vi "GEA_HEWH_SM.vi"(0 "ComPort":refnum<visa-resource-name>="COM1", 1 "Destination Address":u8=96 format="%.0x", 2 "Source Address":u8=128 format="%.0x", 5 "Command":T1=15 items=["RQST_SOFTWARE_VERSION", "RQST_T2_RESISTANCE", "RQST_T3A_RESISTANCE", "RQST_T3B_RESISTANCE", "RQST_T4_RESISTANCE", "RQST_T5_RESISTANCE", "RQST_IDLB_RESISTANCE", "RQST_MODE_SELECT_RESISTANCE", "RQST_DATA_FROM_MEMORY", "RQST_DATA_FROM_DATA_FLASH", "RQST_SS_FAULT_COUNTS", "RQST_OTHER_FAULT_COUNTS", "CMD_CLEAR_FAULT_COUNTS", "RQST_HYPERTERM_OUTPUT_DATA", "CMD_RESET_FILTER_TIMES", "CMD_WRITE_SETPOINTS", "CMD_TURN_ON_OFF_DLB", "CMD_ENTER_EXIT_FCT_MODE", "CMD_SET_LEDS", "CMD_SET_EEV_DRIVE_LINES", "REQ_READ_KEY_STATUS", "RQST_READ_PERSONALITY", "CMD_ENTER_FACT_MODE", "CMD_RESET", "CMD_RESTORE_EEPROM_DEFAULTS", "CMD_SET_MODEL_NUMBER", "CMD_SET_SERIAL_NUMBER", "RQST_MODEL_NUMBER", "RQST_SERIAL_NUMBER", "CMD_TOGGLE_SERVICE_MODE", "CMD_TOGGLE_UE_SERV", "CMD_TOGGLE_LE_SERV", "CMD_REFRESH_SERVICE_TIMEOUTS", "RQST_DSM_OVERRIDE_STATUS", "RQST_STATUS_QUERY", "RQST_HEM_KWH_DATA", "RQST_SERVICE_ERROR_CODES", "RQST_OVERRIDE_STATUS", "CMD_UPDATE_DSM_LEVEL", "CMD_OVERRIDE_STATUS_CHANGED", "CMD_CLEAR_OVERRIDE_STATUS", "CMD_CLEAR_ENERGY_USAGE_CTRS", "CMD_DSM_OVERRIDES", "CMD_UPDATE_MODE", "CMD_SET_PID_P_DENOMINATOR", "CMD_SET_PID_I_DENOM_UNDER_THR", "CMD_SET_PID_I_DENOM_OVER_THR", "CMD_SET_START_POS_UNDER_THR", "CMD_SET_START_POS_OVER_THR", "CMD_SET_EEV_STOP_POSITION", "CMD_SET_AMBIENT_THRESH_1", "CMD_SET_AMBIENT_THRESH_2", "CMD_SET_AMBIENT_THRESH_3", "CMD_SET_PID_LOW_SH_TARGET", "CMD_SET_PID_MID_SH_TARGET", "RQST_PID_PARAMETERS", "CMD_COMP_OFF", "CMD_TOGGLE_FAN", "CMD_RQST_LED_STATUS", "CMD_UE_2_SECONDS", "CMD_LE_2_SECONDS", "CMD_COMP_ON", "CMD_HP_RUN_6MIN", "RQST_TEMP_RANGE", "RQST_VACATION_RANGE", "RQST_STD_ELEC_RANGE", "RQST_WATER_CAPACITY", "CMD_CANCEL_EEV_POSITION", "CMD_EEV_POSITION", "CMD_SET_CURRENTS", "RQST_SUPPORTED_MODES"], 7 "Command Data":u8[](array[numeric]) format="%02x", 9 "InitSerial?":bool=TRUE, 11 "Error In":errorcluster) -> (4 "WriteACK":bool, 6 "Read_ACK":bool, 8 "DataReturned":u8[](array[numeric]) format="%.0x", 14 "CRC Match":bool, 15 "Error Out":errorcluster)   [LabVIEW 2009]
uses:
  HEWH Command Type.ctl
  <vilib>/Instr/_visa.llb/VISA Configure Serial Port (Instr).vi
  HEWH Error Enumeration.ctl
panel:
  out "error out":errorcluster
  out "CRCRead 2":u8[](array[numeric]) format="%.0x"
  out "CRC Calc":u8[](array[numeric]) format="%.0x"
  out "CRCArray":u8[](array[numeric]) format="%.0x"
  out "Destination Read":u8 format="%.0x"
  out "Length":u8
  out "Source Read":u8 format="%.0x"
  out "Partial Message":bool
  out "Current Read Index":i32
  out "byte count":u32=40
  out "Serial Settings:Number of Bytes at Serial Port 3":u32
  out "Serial Settings:Number of Bytes at Serial Port 2":u32
  out "tStart":u32
  out "Tdiff":i32[](array[numeric])
  out "Serial Settings:Number of Bytes at Serial Port":u32
  out "Time Array":i32[](array[numeric])
  out "ACK(E1?)":u8[](array[numeric]) format="%.0x"
  out "Local?":bool
  out "State Array":string[](array[string])
  out "CRCRead":u8[](array[numeric]) format="%.0x"
  out "Command":u8[](array[numeric])=[226, 96, 8, 128, 86, 123, 137, 227] format="%.0x"
  in  "Send HEWH Cmd":bool
  in  "Write Rand":bool
  in  "Random Data":u8[](array[numeric]) format="%.0x"
  out "WriteOK":bool
  out "ReadArray":u8[](array[numeric]) format="%.0x"
  in  "OK":bool
  # "soft version 80,160\nhyerterm data 100,200"
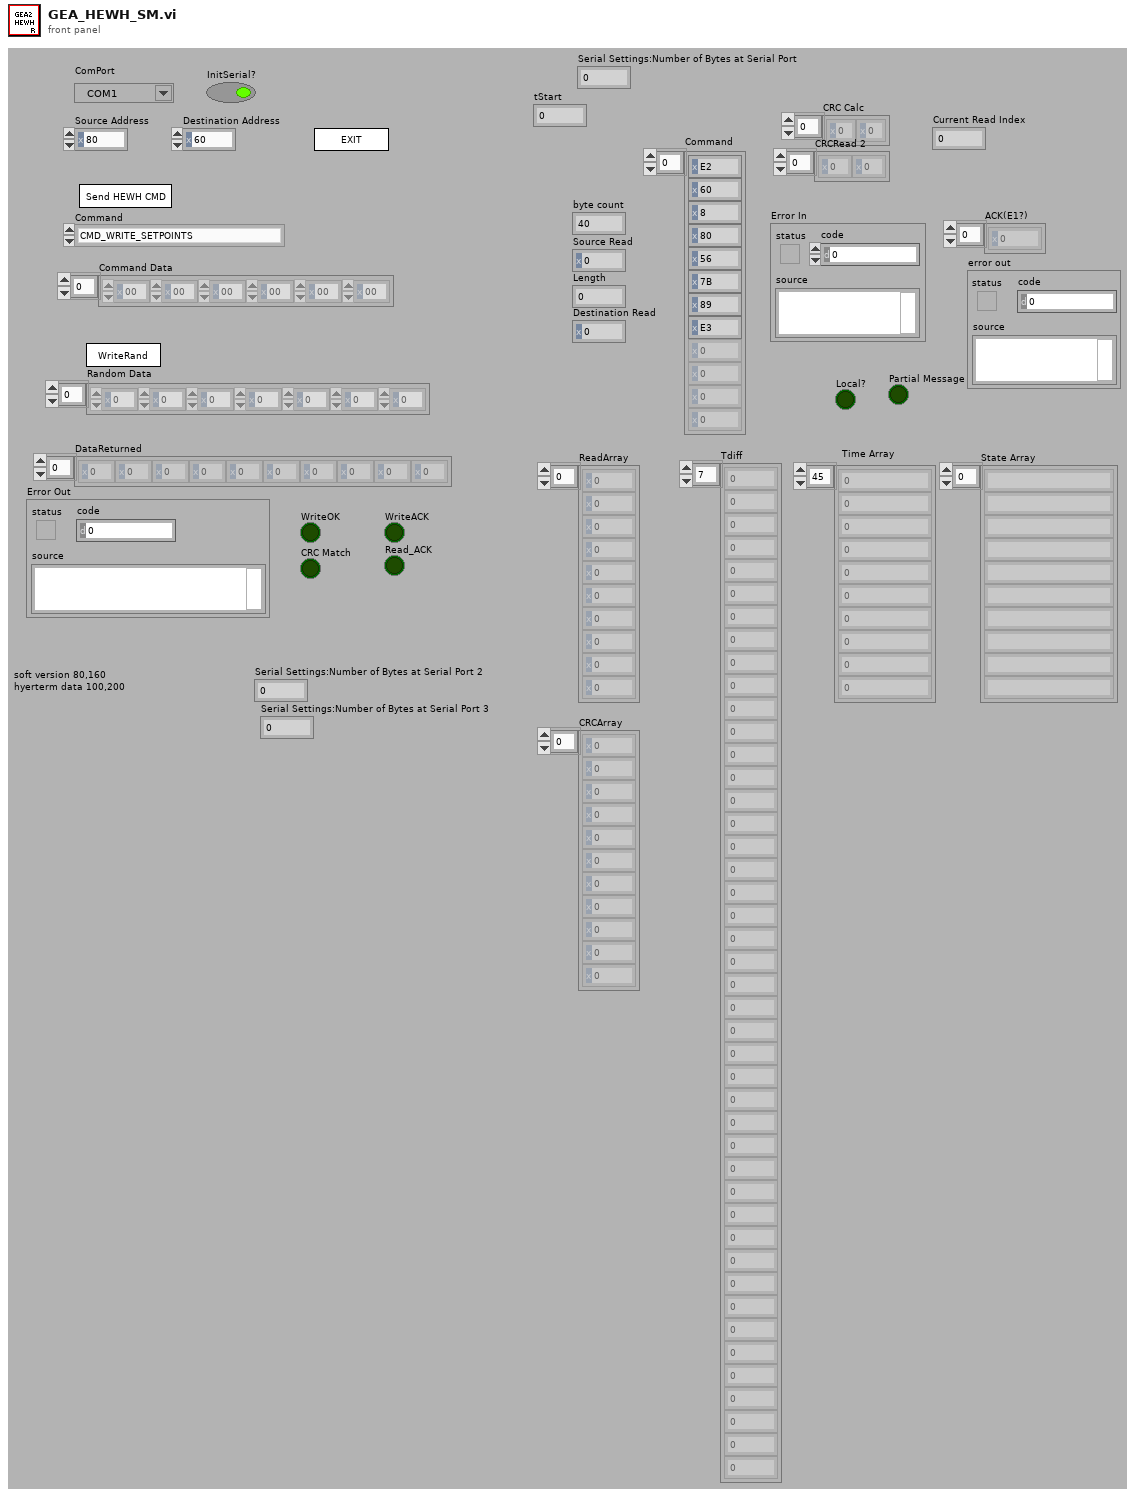
[diagram p1: front panel]
types:
  T1 = typedef "HEWH Command Type.ctl" = u8
  T2 = enum32{"invalid app kind", "Development System", "Run Time System", "Student Edition", "Embedded LabVIEW", "Evaluation", "Custom"}
  T3 = cluster{"Current VI Reference":refnum<vi>, "Close Panel on Exit?":bool}
  T4 = enum32{"Invalid", "Standard", "Closed", "Hidden", "Minimized", "Maximized"}
  T5 = typedef "HEWH Error Enumeration.ctl" = enum16{"No Error", "GEA2 Send ACK Mismatch", "GEA2 STX", "GEA2 ETX", "GEA2 CRC Mismatch", "GEA2 ReadACK", "RTD In Range Error", "Fail Mean Tank Temp", "No Flow Config Data Found", "Failed Flow During Purge", "Temp During Purge", "Confirm IF Stop Fail", "Init Draw: TC_1 Out of Range", "Flow = 0 During Draw after 20s"}
  T6 = cluster{"Core":cluster{"Current VI Reference":refnum<vi>, "Close Panel on Exit?":bool}, "ComPort":refnum<visa-resource-name>, "ReadArray":u8[], "CRCArray":u8[], "Bytes Remaining":u8, "CRCRead":u8[], "CRC":bool, "HEWH Command":u8, "Error Out Flag":bool, "Current Read Index":i32, "Total Bytes Read":u32, "Bytes Data":u8[]}
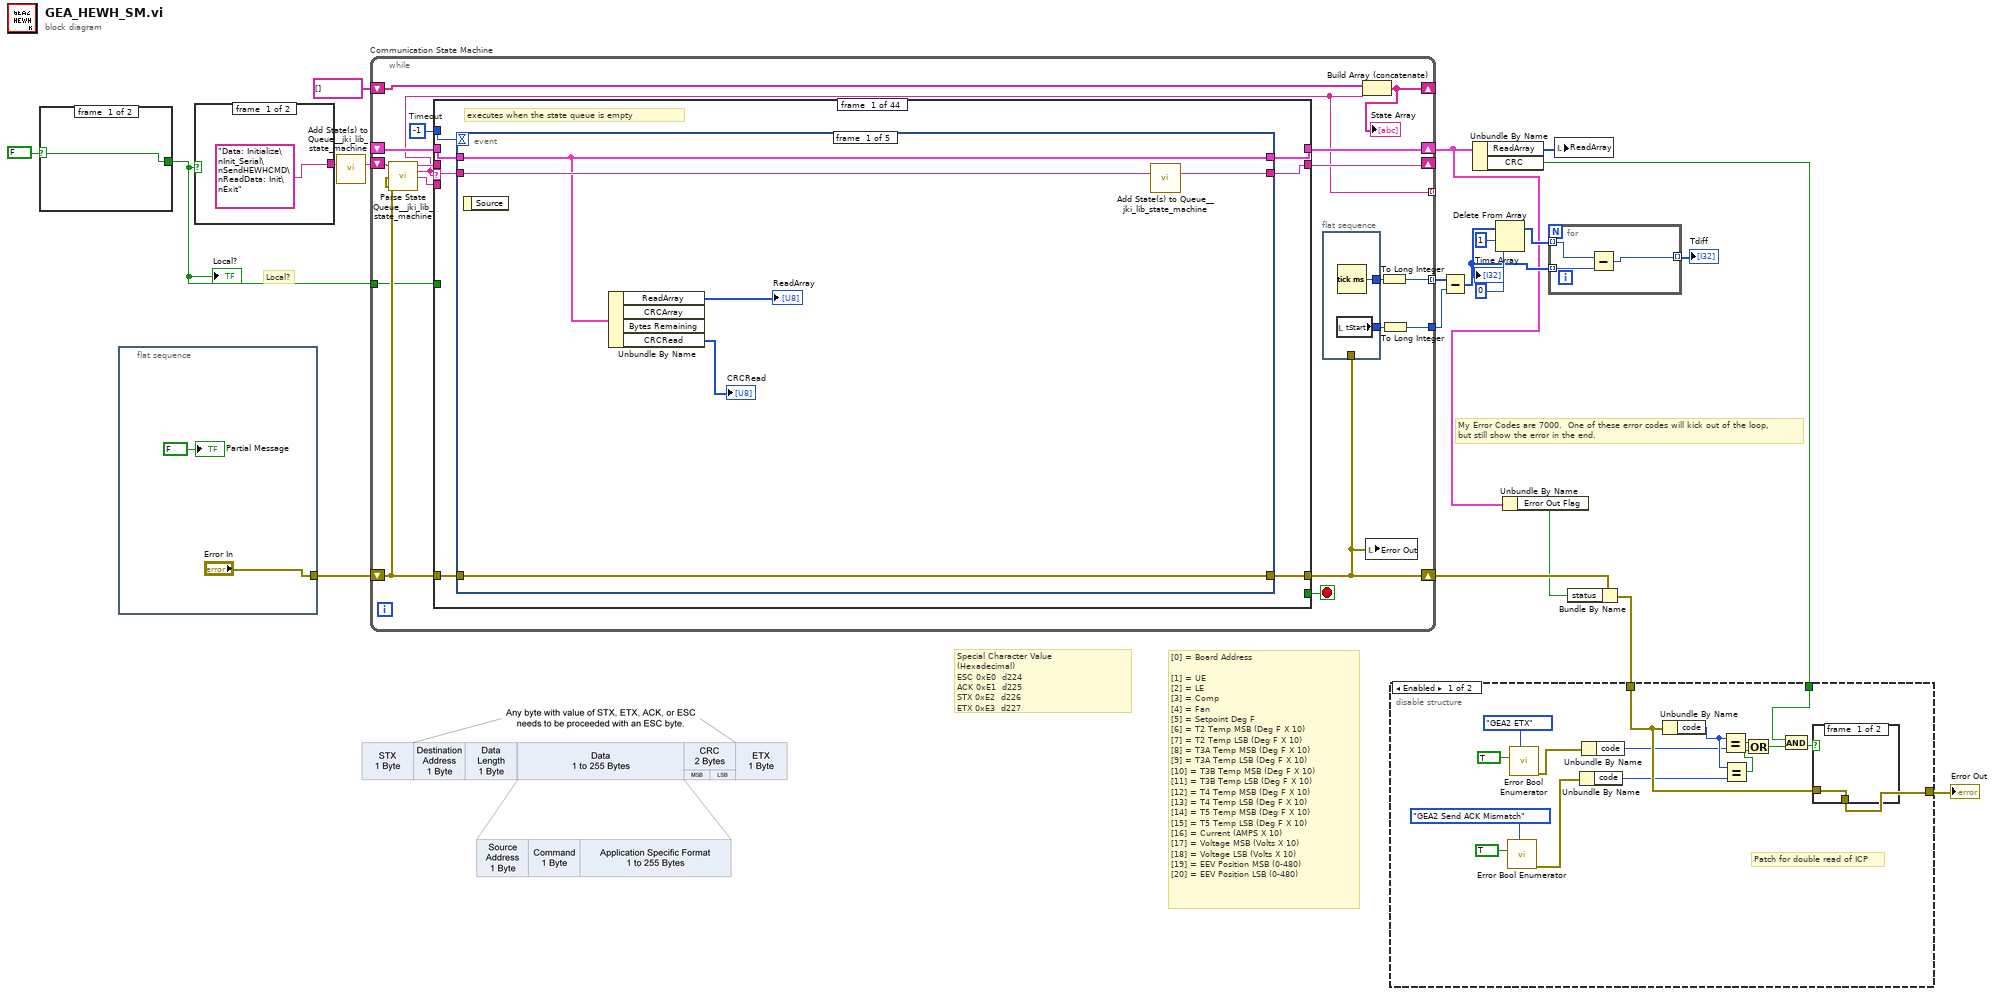
[diagram p0: block diagram]
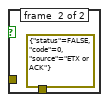
[diagram p2: hidden frame]
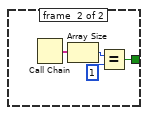
[diagram p4: hidden frame]
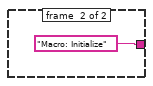
[diagram p5: hidden frame]
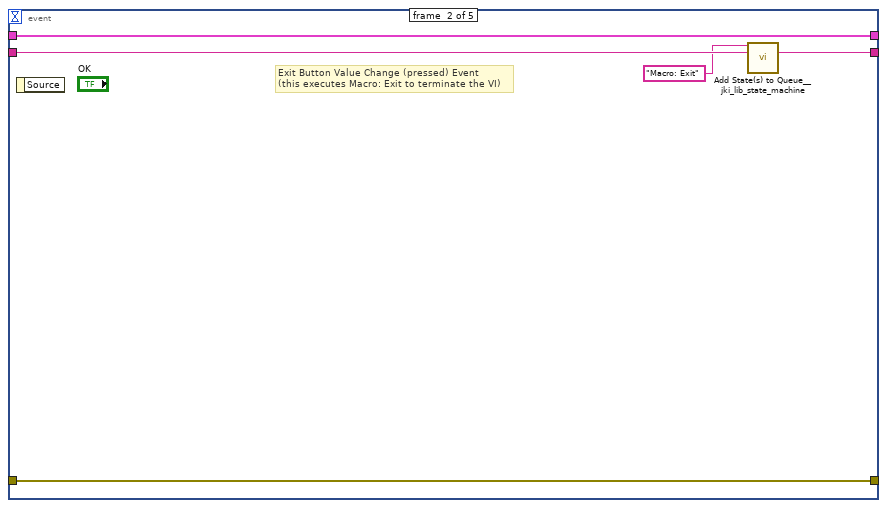
[diagram p6: hidden frame]
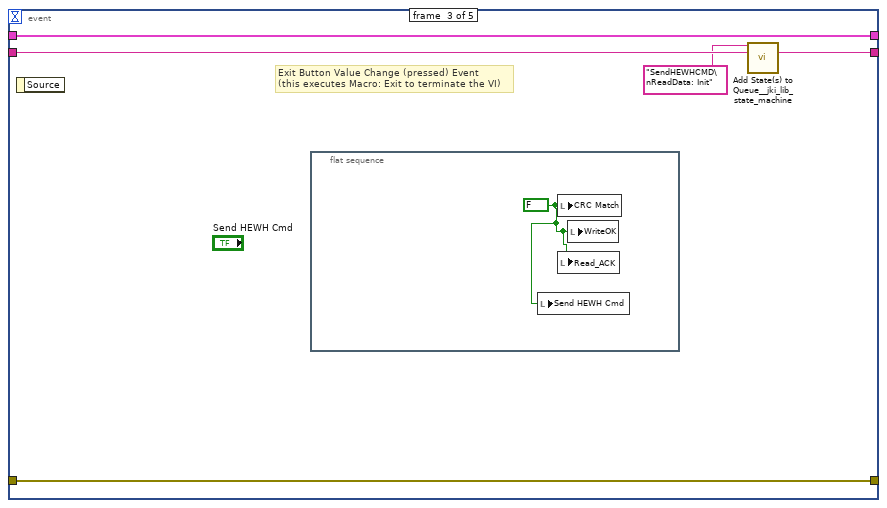
[diagram p7: hidden frame]
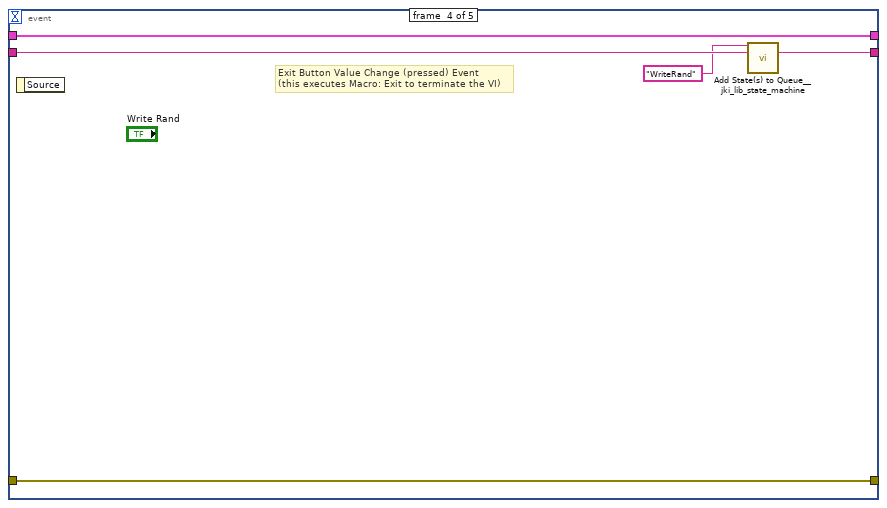
[diagram p8: hidden frame]
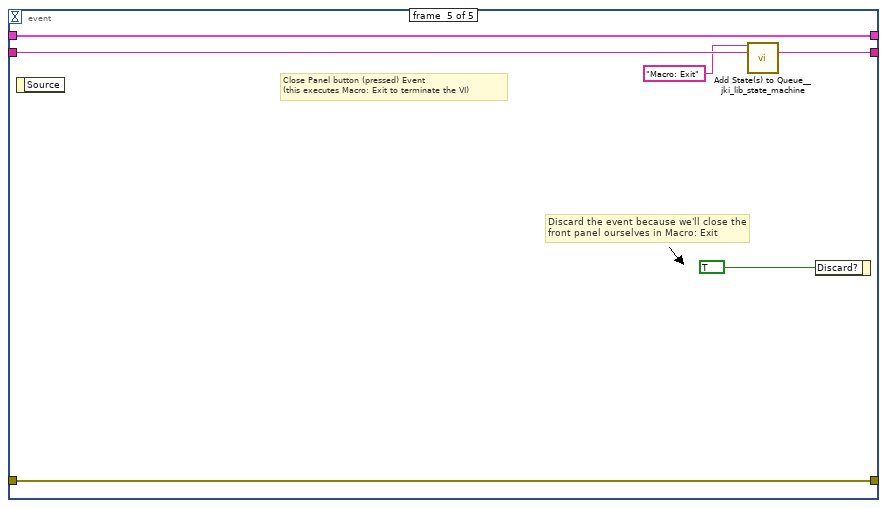
[diagram p9: hidden frame]
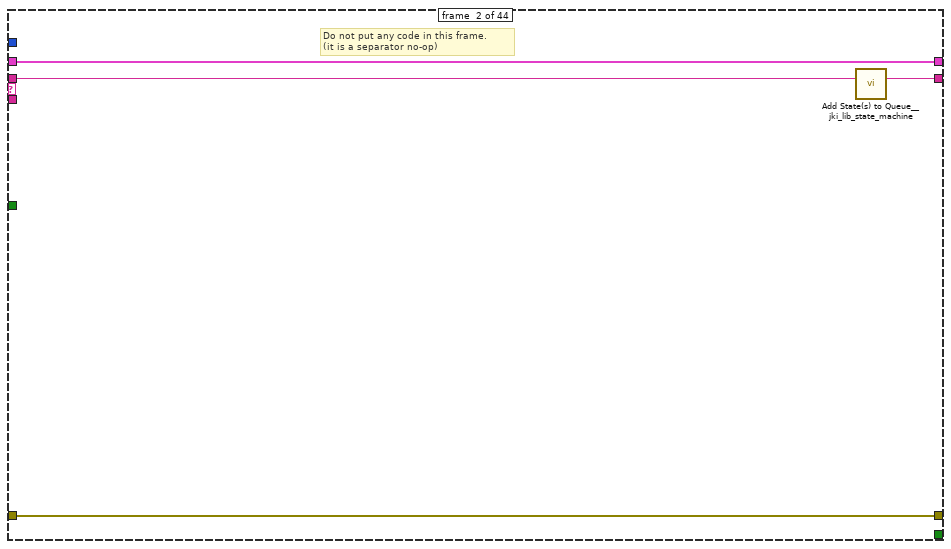
[diagram p10: hidden frame]
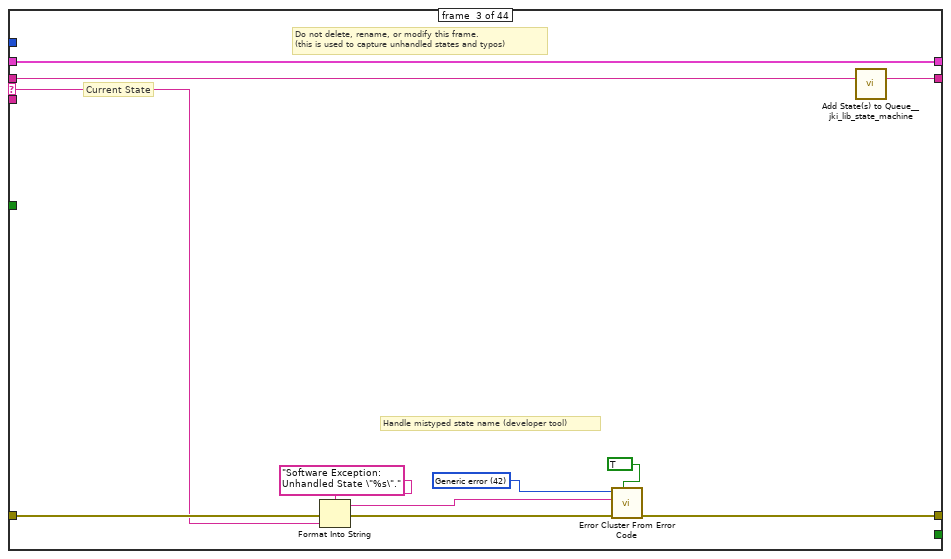
[diagram p11: hidden frame]
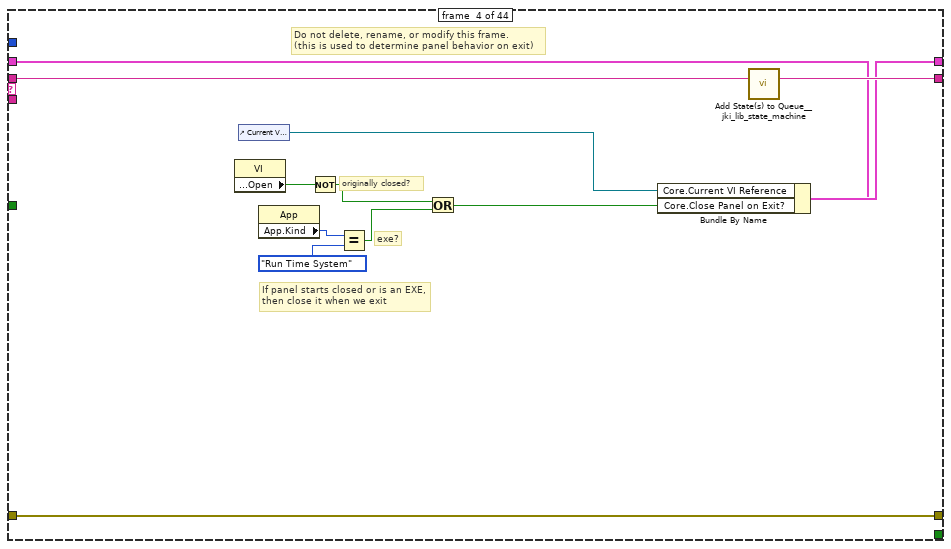
[diagram p12: hidden frame]
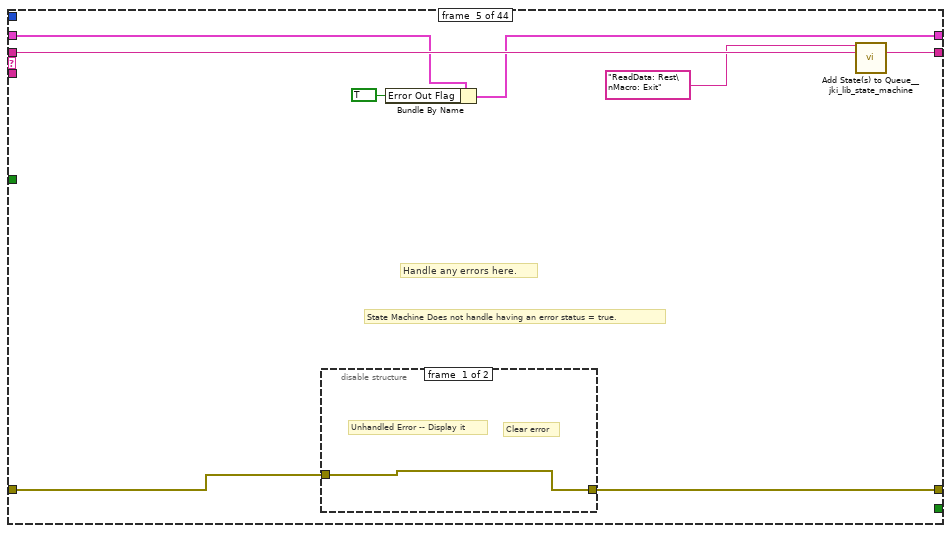
[diagram p13: hidden frame]
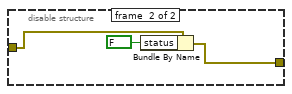
[diagram p14: hidden frame]
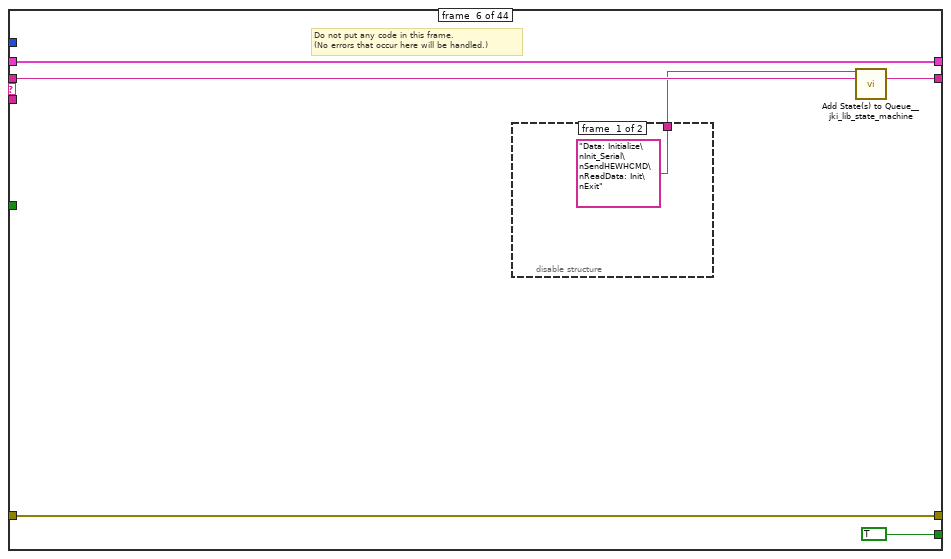
[diagram p15: hidden frame]
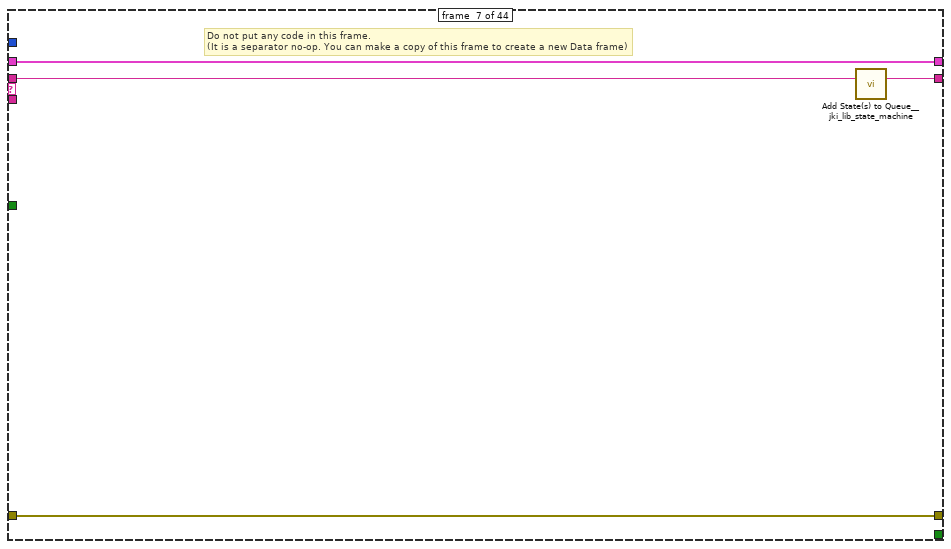
[diagram p17: hidden frame]
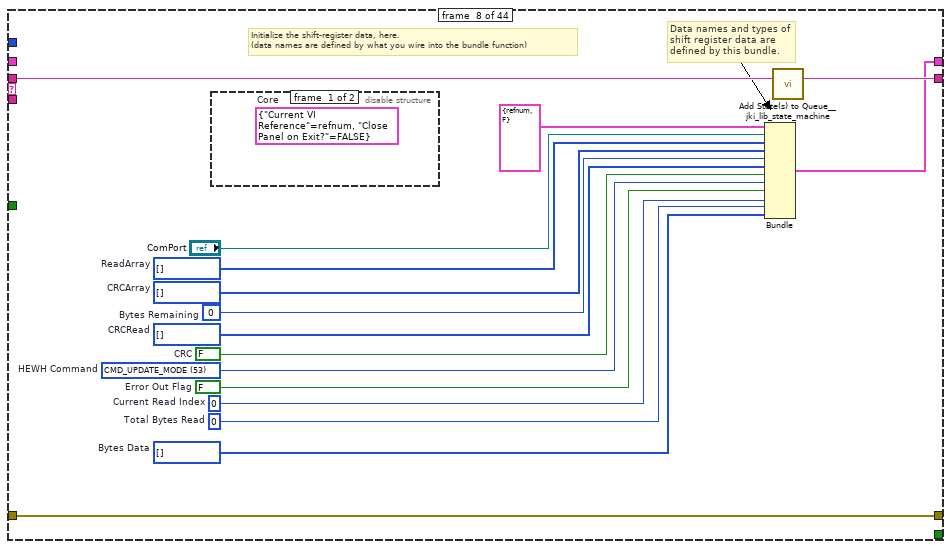
[diagram p18: hidden frame]
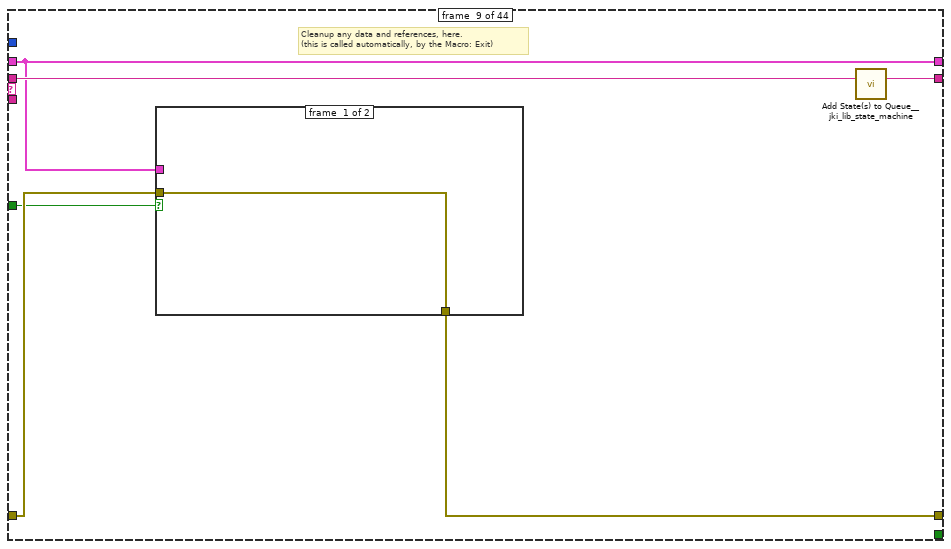
[diagram p20: hidden frame]
diagram:
  # "My Error Codes are 7000.  One of these error codes will kick out of the loop,\nbut still show the error in the end."
  # "Local?"
  # "Special Character\tValue (Hexadecimal)\nESC\t0xE0  d224\nACK\t0xE1  d225\nSTX\t0xE2  d226\nETX\t0xE3  d227"
  # "[0] = Board Address\n\n[1] = UE\n[2] = LE\n[3] = Comp\n[4] = Fan\n[5] = Setpoint Deg F\n[6] = T2 Temp MSB (Deg F X 10)\n[7] = T2 Temp LSB (Deg F X 10)\n[8] = T3A Temp MSB (Deg F X 10)\n[9] = T3A Temp LSB (Deg F X 10)\n[10] = T3B Temp MSB (Deg F X 10)\n[11] = T3B Temp LSB (Deg F X 10)\n[12] = T4 Temp MSB (Deg F X 10)\n[13] = T4 Temp LSB (Deg F X 10)\n[14] = T5 Temp MSB (Deg F X 10)\n[15] = T5 Temp LSB (Deg F X 10)\n[16] = Current (AMPS X 10)\n[17] = Voltage MSB (Volts X 10)\n[18] = Voltage LSB (Volts X 10)\n[19] = EEV Position MSB (0-480)\n[20] = EEV Position LSB (0-480)"
  n1 = case shown="False" FALSE {
    selector: FALSE -> [w21 _]
    tunnel: [w21 w22] -> w17
    frame #0 {
    }
    frame #1 {
      n2 = Call Chain() -> (call chain=w25:string[])
      n3 = Array Size(array=w25) -> (size(s)=w24:i32)
      n4 = Equal?(x=w24, y=1) -> (x = y?=w22:bool)
    }
  }
  "Local?" <- w17
  n5 = flat-sequence {
    tunnel: ["Error In"] -> w18
    frame #0 {
      "Partial Message" <- FALSE ("Partial Message")
    }
  }
  n6 = case shown="False" w17 {
    tunnel: ["Data: Initialize\nInit_Serial\nSendHEWHCMD\nReadData: Init\nExit" "Macro: Initialize"] -> w19
    frame #0 {
    }
    frame #1 {
    }
  }
  n7 = call <vilib>:"Add State(s) to Queue__jki_lib_state_machine.vi"("State(s) in (\"\")"=w19) -> ("States Out"=w20:string)  [unwired: 14 in]
  n8 = while "Communication State Machine" {
    shift-right: [w43] -> w3
    shift-left: _ -> [w42]
    shift-right: [w37] -> w16
    shift-left: w18 -> [w40]
    shift-right: [w38] -> _
    shift-left: w20 -> [w45]
    tunnel: w17 -> [w39]
    tunnel: [w31] -> _ mode=indexing
    tunnel: [w34] -> w10 mode=indexing
    tunnel: [w33] -> w9
    shift-right: [w30] -> _
    shift-left: string[] [] -> [w32]
    stop <- w44 stop-if-true
    w41 = -1  # Timeout
    n9 = call <vilib>:"Parse State Queue__jki_lib_state_machine.vi"("State Queue"=w45, "Error In (no error)"=w40) -> ("Remaining States"=w47:string, "Current State"=w31:string, "Arguments"=w46:string)  [unwired: 11 in]
    n10 = case shown="\"Error Handler\"" w31 {
      selector: w31 -> [_ _ w89 _ _ _ _ _ _ _ _ _ _ _ _ _ _ _ _ _ _ _ _ _ _ _ _ _ _ _ _ _ _ _ _ _ _ _ _ _ _ _ _ _]
      tunnel: w47 -> [w56 w88 w93 w111 w119 w129 w134 w150 w156 w165 w170 w176 w187 w213 w218 w223 w234 w243 w368 w397 w412 w422 w450 w485 w532 w576 w614 w648 w672 w699 w724 w745 w773 w779 w788 w806 w842 w869 w889 w918 w939 w960 w976 w989]
      tunnel: w46 -> [_ _ _ _ _ _ _ _ _ _ _ w171 w181 _ _ _ _ _ _ _ _ _ _ _ _ _ _ _ _ _ _ _ _ _ _ _ _ _ _ _ _ _ _ _]
      tunnel: w42 -> [w54 w85 w91 w102 w114 w127 w131 _ w153 w162 w168 w174 w183 w210 w215 w220 w231 w240 w348 w395 w409 w417 w447 w483 w529 w573 w611 w646 w663 w695 w719 w742 w753 w776 w783 w795 w829 w851 w877 w900 w927 w947 w972 w981]
      tunnel: [w53 w86 w95 w108 w117 w126 w132 w147 w151 w163 w167 w172 w184 w211 w216 w221 w232 w241 w337 w391 w410 w420 w437 w475 w522 w568 w595 w632 w667 w690 w714 w734 w756 w777 w786 w797 w840 w867 w887 w898 w937 w958 w969 w978] -> w37
      tunnel: w40 -> [w52 w86 w94 w108 w116 w126 w132 w147 w154 w163 w167 w173 w185 w211 w216 w221 w232 w238 w334 w392 w410 w420 w440 w477 w524 w569 w607 w642 w669 w693 w717 w733 w771 w777 w786 w798 w840 w867 w887 w898 w937 w958 w970 w979]
      tunnel: [w55 w87 w92 w110 w118 w128 w133 w149 w155 w164 w169 w175 w186 w212 w217 w222 w233 w242 w367 w396 w411 w421 w449 w484 w531 w575 w613 w647 w671 w698 w723 w744 w772 w778 w787 w805 w841 w868 w888 w917 w938 w959 w975 w988] -> w38
      tunnel: [_ _ _ _ _ TRUE _ _ _ _ _ _ _ _ _ _ _ _ _ _ _ _ _ _ _ _ _ _ _ _ _ _ _ _ _ _ _ _ _ _ _ _ _ _] -> w44
      tunnel: [w51 w85 w91 w109 w113 w127 w131 w148 w153 w162 w168 w174 w183 w210 w215 w220 w231 w239 w347 w395 w409 w419 w446 w482 w528 w572 w610 w645 w662 w694 w718 w741 w752 w776 w785 w794 w828 w850 w876 w899 w926 w946 w971 w980] -> w43
      tunnel: w41 -> [w50 _ _ _ _ _ _ _ _ _ _ _ _ _ _ _ _ _ _ _ _ _ _ _ _ _ _ _ _ _ _ _ _ _ _ _ _ _ _ _ _ _ _ _]
      tunnel: w39 -> [_ _ _ _ _ _ _ _ w152 _ _ _ _ _ _ _ _ w237 _ _ _ _ _ _ _ _ _ _ _ _ _ _ _ _ _ _ _ _ _ _ _ _ _ _]
      frame #0 {
        # "executes when the state queue is empty"
        n11 = event shown="[4] Panel Close?" {
          selector: _ -> [_ _ _ _ _]
          dyn-events: _ -> [_ _ _ _ _]
          timeout: w50 -> [_ _ _ _ _]
          tunnel: w56 -> [w62 w67 w72 w78 w84]
          tunnel: [w61 w66 w71 w77 w83] -> w55
          tunnel: w54 -> [w59 w64 w69 w75 w81]
          tunnel: [w60 w65 w70 w76 w82] -> w53
          tunnel: w52 -> [w60 w65 w70 w76 w82]
          tunnel: [w59 w64 w69 w75 w81] -> w51
          event #0 {
            n12 = event-data() -> ()  [unwired: 1 in, 1 out]
            n13 = Unbundle By Name(w59) -> ("ReadArray"=→"ReadArray":u8[], "CRCRead"=→"CRCRead":u8[])  [unwired: 2 out]
            n14 = call <vilib>:"Add State(s) to Queue__jki_lib_state_machine.vi"("State(s) in (\"\")"=w62) -> ("States Out"=w61:string)  [unwired: 14 in]
          }
          event #1 {
            # "Exit Button Value Change (pressed) Event\n(this executes Macro: Exit to terminate the VI)"
            n15 = event-data() -> ()  [unwired: 1 in, 1 out]
            n16 = call <vilib>:"Add State(s) to Queue__jki_lib_state_machine.vi"("State(s) in Front (\"\")"="Macro: Exit", "State(s) in (\"\")"=w67) -> ("States Out"=w66:string)  [unwired: 13 in]
          }
          event #2 {
            # "Exit Button Value Change (pressed) Event\n(this executes Macro: Exit to terminate the VI)"
            n17 = event-data() -> ()  [unwired: 1 in, 1 out]
            n18 = flat-sequence {
              frame #0 {
                w73 = FALSE ("CRC Match")
                n19 = local write "Send HEWH Cmd"(w73) -> ()
                n20 = local write "CRC Match"(w73) -> ()
                n21 = local write "Read_ACK"(w73) -> ()
                n22 = local write "WriteOK"(w73) -> ()
              }
            }
            n23 = call <vilib>:"Add State(s) to Queue__jki_lib_state_machine.vi"("State(s) in Front (\"\")"="SendHEWHCMD\nReadData: Init", "State(s) in (\"\")"=w72) -> ("States Out"=w71:string)  [unwired: 13 in]
          }
          event #3 {
            # "Exit Button Value Change (pressed) Event\n(this executes Macro: Exit to terminate the VI)"
            n24 = event-data() -> ()  [unwired: 1 in, 1 out]
            n25 = call <vilib>:"Add State(s) to Queue__jki_lib_state_machine.vi"("State(s) in Front (\"\")"="WriteRand", "State(s) in (\"\")"=w78) -> ("States Out"=w77:string)  [unwired: 13 in]
          }
          event #4 {
            # "Discard the event because we'll close the front panel ourselves in Macro: Exit"
            # "Close Panel button (pressed) Event\n(this executes Macro: Exit to terminate the VI)"
            n26 = event-data() -> ()  [unwired: 1 in, 1 out]
            n27 = call <vilib>:"Add State(s) to Queue__jki_lib_state_machine.vi"("State(s) in Front (\"\")"="Macro: Exit", "State(s) in (\"\")"=w84) -> ("States Out"=w83:string)  [unwired: 13 in]
            n28 = event-data("Discard?"=TRUE) -> ()  [unwired: 1 in, 1 out]
          }
        }
      }
      frame #1 {
        # "Do not put any code in this frame.\n(it is a separator no-op)"
        n29 = call <vilib>:"Add State(s) to Queue__jki_lib_state_machine.vi"("State(s) in (\"\")"=w88) -> ("States Out"=w87:string)  [unwired: 14 in]
      }
      frame #2 {
        w98 = 42 items=["No error", "Argument error", "Memory is full", "Out of zone", "End of file", "File already open", "Generic file I/O error", "File not found", "File permission error", "Disk is full", "Duplicate path", "Too many files open", "System feature not enabled", "Resource file not found", "Cannot add resource", "Resource not found", "Image not found", "Image memory error", "Pen does not exist", "Config type invalid", "Config token not found", "Config parse error", "Config memory error", "Bad external code format", "Bad external code offset", "External code not present", "Null window", "Destroy window error", "Null menu", "Print aborted", "Bad print record", "Print driver error", "Windows error during printing", "Memory error during printing", "Print dialog error", "Generic print error", "Invalid device refnum", "Device not found", "Device parameter error", "Device unit error", "Cannot open device", "Device call aborted", "Generic error", "Cancelled by user", "Object ID too low", "Object ID too high", "Object not in heap", "Unknown heap", "Unknown object (invalid DefProc)", "Unknown object (DefProc not in table)", "Message out of range", "Invalid (null) method", "Unknown message", "Manager call not supported", "Bad address", "Network operation in progress", "Network operation timed out", "Connection is busy", "Network attribute not supported", "Network error", "Address in use", "System out of memory", "Connection aborted", "Connection refused", "Not connected", "Already connected", "Connection closed", "Initialization error (interapplication manager)", "Bad occurrence", "Wait on unbound occurrence handler", "Occurrence queue overflow", "Datalog type conflict", "Unused", "Unrecognized type (interapplication manager)", "Memory corrupt", "Failed to make temporary DLL", "Old CIN version", "Drag socket not found", "Failed to load drop-object", "Failed to register OLE object", "Failed to release OLE object", "Format specifier type mismatch", "Unknown format specifier", "Too few format specifiers", "Too many format specifiers", "Scan failed", "Newer CIN version", "Error converting to variant", "Runtime menu error", "Password tampered", "Variant attribute not found", "Incompatible variant data type", "Event data is not available", "Event Store is not present", "Occurrence is not found", "Event Queue is not created", "Event info is not available", "Refnum passed is NULL", "Error retrieving Class GUID", "Error retrieving CoClass GUID", "Error retrieving TypeLib GUID.", "Bad built application magic bytes.", "Specific driver is different from the specific driver associated with the Logical Name.", "There is no session opened to the class driver.", "Max Error", "MAX - Error with config objects", "MAX - Error loading configuration", "MAX - Group not supported"]
        # "Current State"
        # "Do not delete, rename, or modify this frame.\n(this is used to capture unhandled states and typos)"
        # "Handle mistyped state name (developer tool)"
        n30 = Format Into String(format string="Software Exception: Unhandled State \"%s\"." ("message"), error in=w94, w89) -> (resulting string=w97:string, error out=w96:errorcluster)  [unwired: 1 in]
        n31 = call <vilib>:"Error Cluster From Error Code.vi"("show call chain? (False)"=TRUE, "error in (no error)"=w96, "error message (\"\")"=w97, "error code (0)"=w98) -> ("error out"=w95:errorcluster)  [unwired: 5 in]
        n32 = call <vilib>:"Add State(s) to Queue__jki_lib_state_machine.vi"("State(s) in (\"\")"=w93) -> ("States Out"=w92:string)  [unwired: 14 in]
      }
      frame #3 {
        # "Do not delete, rename, or modify this frame.\n(this is used to determine panel behavior on exit)"
        # "originally closed?"
        # "exe?"
        # "If panel starts closed or is an EXE, then close it when we exit"
        n33 = property class="VI"() -> ("Front Panel.Open"=w107:bool)  [unwired: 2 in, 2 out]
        n34 = control-ref of="Current VI Reference"() -> (w100:refnum<vi>)
        n35 = property class="App"() -> ("App.Kind"=w106:T2)  [unwired: 2 in, 2 out]
        n36 = Not(x=w107) -> (.not. x?=w104:bool)
        n37 = Equal?(x=w106, y=T2."Run Time System" ("Application:Kind")) -> (x = y?=w103:bool)
        n38 = Or(x=w104, y=w103) -> (x .or. y?=w101:bool)
        n39 = Bundle By Name(cluster=w102, "Core.Current VI Reference"=w100, "Core.Close Panel on Exit?"=w101) -> (w109:T6)
        n40 = call <vilib>:"Add State(s) to Queue__jki_lib_state_machine.vi"("State(s) in (\"\")"=w111) -> ("States Out"=w110:string)  [unwired: 14 in]
      }
      frame #4 {
        # "State Machine Does not handle having an error status = true."
        # "Handle any errors here."
        n41 = disable-structure shown="Enabled" {
          disable-tunnel: [w120 w122] -> w117
          disable-tunnel: w116 -> [w120 w123]
          frame #0 {
            # "Unhandled Error -- Display it"
            # "Clear error"
          }
          frame #1 {
            n42 = Bundle By Name(cluster=w123, "status"=FALSE) -> (w122:errorcluster)
          }
        }
        n43 = Bundle By Name(cluster=w114, "Error Out Flag"=TRUE) -> (w113:T6)
        n44 = call <vilib>:"Add State(s) to Queue__jki_lib_state_machine.vi"("State(s) in Front (\"\")"="ReadData: Rest\nMacro: Exit", "State(s) in (\"\")"=w119) -> ("States Out"=w118:string)  [unwired: 13 in]
      }
      frame #5 {
        # "Do not put any code in this frame.\n(No errors that occur here will be handled.)"
        n45 = disable-structure shown="Enabled" {
          disable-tunnel: ["Data: Initialize\nInit_Serial\nSendHEWHCMD\nReadData: Init\nExit" _] -> w124
          frame #0 {
          }
          frame #1 {
          }
        }
        n46 = call <vilib>:"Add State(s) to Queue__jki_lib_state_machine.vi"("State(s) in Front (\"\")"=w124, "State(s) in (\"\")"=w129) -> ("States Out"=w128:string)  [unwired: 13 in]
      }
      frame #6 {
        # "Do not put any code in this frame.\n(It is a separator no-op. You can make a copy of this frame to create a new Data frame)"
        n47 = call <vilib>:"Add State(s) to Queue__jki_lib_state_machine.vi"("State(s) in (\"\")"=w134) -> ("States Out"=w133:string)  [unwired: 14 in]
      }
      frame #7 {
        w135 = u8[] []  # Bytes Data
        w136 = u32 0  # Total Bytes Read
        w137 = 0  # Current Read Index
        w138 = FALSE  # Error Out Flag
        w139 = u8 53 items=["CMD_WRITE_SETPOINTS", "RQST_NON_CRIT_VERSION", "RQST_CRIT_VERSION", "RQST_EEPROM_VERSION", "RQST_T2_RESISTANCE", "RQST_T3A_RESISTANCE", "RQST_T3B_RESISTANCE", "RQST_T4_RESISTANCE", "RQST_T5_RESISTANCE", "RQST_IDLB_RESISTANCE", "RQST_MODE_SELECT_RESISTANCE", "RQST_STATUS INFO", "RQST_SS_FAULT_COUNTS", "RQST_OTHER_FAULT_COUNTS", "CMD_CLEAR_FAULT_COUNTS", "RQST_HYPERTERM_OUTPUT_DATA", "RQST_READ_PERSONALITY", "RQST_DSM_OVERRIDE_STATUS", "RQST_STATUS_QUERY", "RQST_HEM_KWH_DATA", "RQST_SERVICE_ERROR_CODES", "RQST_OVERRIDE_STATUS", "CMD_CLEAR_OVERRIDE_STATUS", "CMD_CLEAR_ENERGY_USAGE_CTRS", "CMD_COMP_OFF", "CMD_UE_2_SECONDS", "CMD_LE_2_SECONDS", "CMD_COMP_ON", "CMD_HP_RUN_6MIN", "RQST_TEMP_RANGE", "RQST_VACATION_RANGE", "RQST_STD_ELEC_RANGE", "RQST_WATER_CAPACITY", "CMD_CANCEL_EEV_POSITION", "RQST_SUPPORTED_MODES", "CMD_CONTROL_FAN1", "CMD_EEV_POSITION", "CMD_SET_EEV_START_POSITION", "CMD_SET_EEV_STOP_POSITION", "CMD_UPDATE_DSM_LEVEL", "CMD_SET_PID_I_DENOMINATOR", "CMD_SET_PID_I_NUMERATOR", "RQST_DATA_FROM_MEMORY", "CMD_OVERRIDE_STATUS_CHANGED", "CMD_SET_PID_P_DENOMINATOR", "CMD_SET_PID_P_NUMERATOR", "CMD_SET_PID_RUN_SH_TARGET", "CMD_SET_PID_START_DWELL_TIME", "CMD_SET_PID_TRANSITION_TIME", "CMD_SET_PID_TRANS_SH_TARGET", "CMD_SET_PID_UPDATE_RATE", "RQST_DATA_FROM_DATA_FLASH", "CMD_DSM_OVERRIDES", "CMD_UPDATE_MODE", "CMD_UPDATE_SPECIAL_OPERATION", "CMD_SET_CURRENTS", "CMD_RESET_FILTER_TIMES", "CMD_TURN_ON_DLB", "RQST_PID_PARAMETERS", "CMD_CHECK_CRC", "CMD_ENTER_FACT_MODE", "CMD_RESET", "CMD_RESTORE_EEPROM_DEFAULTS"]  # HEWH Command
        w141 = FALSE  # CRC
        w142 = u8[] []  # CRCRead
        w143 = u8 0  # Bytes Remaining
        w144 = u8[] []  # CRCArray
        w145 = u8[] []  # ReadArray
        # "Data names and types of shift register data are defined by this bundle."
        # "Initialize the shift-register data, here.\n(data names are defined by what you wire into the bundle function)"
        n48 = disable-structure shown="Enabled" {
          frame #0 {
            (unwired) T3 {"Current VI Reference"=refnum, "Close Panel on Exit?"=FALSE}  # Core
          }
          frame #1 {
          }
        }
        n49 = Bundle("Core"=T3 {"Current VI Reference"=refnum, "Close Panel on Exit?"=FALSE}, "ComPort"="ComPort", "ReadArray"=w145, "CRCArray"=w144, "Bytes Remaining"=w143, "CRCRead"=w142, "CRC"=w141, "HEWH Command"=w139, "Error Out Flag"=w138, "Current Read Index"=w137, "Total Bytes Read"=w136, "Bytes Data"=w135) -> (w148:T6)  [unwired: 1 in]
        n50 = call <vilib>:"Add State(s) to Queue__jki_lib_state_machine.vi"("State(s) in (\"\")"=w150) -> ("States Out"=w149:string)  [unwired: 14 in]
      }
      frame #8 {
        # "Cleanup any data and references, here.\n(this is called automatically, by the Macro: Exit)"
        n51 = case shown="True" w152 {
          tunnel: w154 -> [w157 w160]
          tunnel: [w157 w159] -> w151
          tunnel: w153 -> [_ w158]
          frame #0 {
          }
          frame #1 {
            n52 = Unbundle By Name(w158) -> ("Core.Current VI Reference"=w161:refnum<vi>)
            n53 = Close Reference(reference=w161, error in (no error)=w160) -> (error out=w159:errorcluster)
          }
        }
        n54 = call <vilib>:"Add State(s) to Queue__jki_lib_state_machine.vi"("State(s) in (\"\")"=w156) -> ("States Out"=w155:string)  [unwired: 14 in]
      }
      frame #9 {
        # "Do not put any code in this frame.\n(It is a separator no-op. You can make a copy of this frame to create a new UI frame)"
        n55 = call <vilib>:"Add State(s) to Queue__jki_lib_state_machine.vi"("State(s) in (\"\")"=w165) -> ("States Out"=w164:string)  [unwired: 14 in]
      }
      frame #10 {
        w166 = FALSE ("CRC Match")
        # "Initialize the User Interface, here.\n(this is called automatically, by the Macro: Init)"
        n56 = local write "CRC Match"(w166) -> ()
        n57 = local write "WriteOK"(w166) -> ()
        n58 = local write "WriteACK"(w166) -> ()
        n59 = local write "Send HEWH Cmd"(w166) -> ()
        n60 = call <vilib>:"Add State(s) to Queue__jki_lib_state_machine.vi"("State(s) in (\"\")"=w170) -> ("States Out"=w169:string)  [unwired: 14 in]
      }
      frame #11 {
        # "Argument"
        # "Set and Unset Cursor Busy.\n(Usage: \"UI: Cursor Set >> Busy|Idle\")"
        n61 = case shown="\"Idle\", Default" w171 {
          tunnel: w173 -> [w178 w180]
          tunnel: [w177 w179] -> w172
          frame #0 {
            n62 = call <vilib>:"Unset Busy.vi"("error in (no error)"=w178) -> ("error out"=w177:errorcluster)  [unwired: 10 in]
          }
          frame #1 {
            n63 = call <vilib>:"Set Busy.vi"("error in (no error)"=w180) -> ("error out"=w179:errorcluster)  [unwired: 9 in, 1 out]
          }
        }
        n64 = call <vilib>:"Add State(s) to Queue__jki_lib_state_machine.vi"("State(s) in (\"\")"=w176) -> ("States Out"=w175:string)  [unwired: 14 in]
      }
      frame #12 {
        # "Argument"
        # "Set Front Panel Open or Closed\n(Usage: \"UI: Front Panel State >> Open|Close\")"
        n65 = Unbundle By Name(w183) -> ("Core.Current VI Reference"=w182:refnum<vi>)
        n66 = case shown="\"Close\"" w181 {
          tunnel: w185 -> [w191 w204]
          tunnel: [w193 w205] -> w184
          tunnel: w182 -> [w192 w202]
          frame #0 {
            n67 = property class="VI"(reference=w192, error in=w191) -> (reference out=w189:refnum<vi>, error out=w190:errorcluster, "Front Panel.Open"=w188:bool)
            n68 = case shown="False" w188 {
              tunnel: [w196 w199] -> w193
              tunnel: w190 -> [w195 w199]
              tunnel: w189 -> [w194 _]
              frame #0 {
                n69 = invoke class="VI" method="FP.Open"(reference=w194, error in=w195, "Activate"=TRUE, "State"=T4."Standard") -> (error out=w196:errorcluster)  [unwired: 1 in, 4 out]
              }
              frame #1 {
              }
            }
          }
          frame #1 {
            n70 = property class="VI"(reference=w202, error in=w204) -> (reference out=w201:refnum<vi>, error out=w203:errorcluster, "Front Panel.Open"=w200:bool)
            n71 = case shown="True" w200 {
              tunnel: [w206 w209] -> w205
              tunnel: w203 -> [w206 w208]
              tunnel: w201 -> [_ w207]
              frame #0 {
              }
              frame #1 {
                n72 = invoke class="VI" method="FP.Close"(reference=w207, error in=w208) -> (error out=w209:errorcluster)  [unwired: 1 in, 2 out]
              }
            }
          }
        }
        n73 = call <vilib>:"Add State(s) to Queue__jki_lib_state_machine.vi"("State(s) in (\"\")"=w187) -> ("States Out"=w186:string)  [unwired: 14 in]
      }
      frame #13 {
        # "Do not put any code in this frame.\n(It is a separator no-op. You can make a copy of this frame to create a new Macro frame)"
        n74 = call <vilib>:"Add State(s) to Queue__jki_lib_state_machine.vi"("State(s) in (\"\")"=w213) -> ("States Out"=w212:string)  [unwired: 14 in]
      }
      frame #14 {
        w214 = "Data: Initialize\nInitialize Core Data\nUI: Initialize\nUI: Front Panel State >> Open\nInit_Serial"  # Data: Initialize Initialize Core Data UI: Initialize UI: Front Panel State >> Open Init_Serial
        # "Initialization Macro\n(This is called once, when the VI starts)"
        n75 = call <vilib>:"Add State(s) to Queue__jki_lib_state_machine.vi"("State(s) in Front (\"\")"=w214, "State(s) in (\"\")"=w218) -> ("States Out"=w217:string)  [unwired: 13 in]
      }
      frame #15 {
        # "Exit Macro\n(This is called once, when the VI exits)"
        n76 = disable-structure shown="Enabled" {
          disable-tunnel: w220 -> [w230 _]
          disable-tunnel: [w224 _] -> w219
          frame #0 {
            n77 = Unbundle By Name(w230) -> ("Core.Close Panel on Exit?"=w229:bool)
            n78 = Select(t="UI: Front Panel State >> Close", s=w229, f="") -> (s? t:f=w226:string)
            n79 = call <vilib>:"Add State(s) to Queue__jki_lib_state_machine.vi"("State(s) in (\"\")"=w226, "State(s) at Back (\"\")"="Data: Cleanup\nExit") -> ("States Out"=w224:string)  [unwired: 13 in]
          }
          frame #1 {
          }
        }
        n80 = call <vilib>:"Add State(s) to Queue__jki_lib_state_machine.vi"("State(s) in Front (\"\")"=w219, "State(s) in (\"\")"=w223) -> ("States Out"=w222:string)  [unwired: 13 in]
      }
      frame #16 {
        # "Template Separator\n(You can make a copy of, or modify, this frame)"
        n81 = call <vilib>:"Add State(s) to Queue__jki_lib_state_machine.vi"("State(s) in (\"\")"=w234) -> ("States Out"=w233:string)  [unwired: 14 in]
      }
      frame #17 {
        # "Your code here.\n(You can make a copy of, or modify, this frame)"
        n82 = case shown="True" "InitSerial?" {
          tunnel: [w248 w270] -> w241
          tunnel: w240 -> [w247 w280]
          tunnel: [w246 w279] -> w239
          tunnel: w238 -> [w253 w273]
          tunnel: w237 -> [_ _]
          tunnel: [w245 w271] -> w235
          frame #0 {
            # "skip error handle routine"
            n83 = Unbundle By Name(w247) -> ("ComPort"=w244:refnum<visa-resource-name>)
            n84 = property class="Instr"(reference=w244) -> (reference out=w250:refnum<visa-resource-name>, "Serial Settings:Number of Bytes at Serial Port"=w252:u32)  [unwired: 1 in, 1 out]
            n85 = Greater Than 0?(x=w252) -> (x > 0?=w251:bool)
            n86 = case shown="True" w251 {
              tunnel: w253 -> [w266 w269]
              tunnel: [w266 w268] -> w249
              tunnel: w250 -> [_ w267]
              frame #0 {
              }
              frame #1 {
                n87 = VISA Clear(VISA resource name=w267, error in (no error)=w269) -> (error out=w268:errorcluster)  [unwired: 1 out]
              }
            }
            n88 = case shown="No Error" w249 {
              selector: w249 -> [w254 w261]
              tunnel: w247 -> [w258 w265]
              tunnel: [w257 w264] -> w246
              tunnel: w244 -> [w256 _]
              tunnel: ["" ("State(s) in Front (\"\")") "Macro: Exit" ("State(s) in Front (\"\")")] -> w245
              tunnel: [w254 w260] -> w248
              frame #0 {
                n89 = Bundle By Name(cluster=w258, "ComPort"=w256) -> (w257:T6)
              }
              frame #1 {
                n90 = Bundle By Name(cluster=w265, "Error Out Flag"=TRUE) -> (w264:T6)
                n91 = Bundle By Name(cluster=w261, "status"=FALSE) -> (w260:errorcluster)
              }
            }
          }
          frame #1 {
            # "skip error handle routine"
            # "Assumes that if the serial port is 19200, then it is all ok."
            n92 = Unbundle By Name(w280) -> ("ComPort"=w278:refnum<visa-resource-name>)
            n93 = disable-structure shown="Enabled" {
              disable-tunnel: w278 -> [w316 _]
              disable-tunnel: [w313 TRUE] -> w277
              frame #0 {
                n94 = property class="Instr"(reference=w316) -> ("Baud"=w315:u32)  [unwired: 1 in, 2 out]
                n95 = Not Equal?(x=w315, y=u32 19200) -> (x != y?=w313:bool)
              }
              frame #1 {
              }
            }
            n96 = case shown="True" w277 {
              tunnel: [w318 w321] -> w276
              tunnel: [w319 w320] -> w274
              tunnel: w273 -> [w318 w323]
              tunnel: w278 -> [w319 w322]
              frame #0 {
              }
              frame #1 {
                w329 = u16 0 items=["None", "XON/XOFF", "RTS/CTS", "XON/XOFF & RTS/CTS", "DTR/DSR", "XON/XOFF & DTR/DSR"] ("flow control (0:none)")
                w328 = u16 10 items=["1.0"=10, "1.5"=15, "2.0"=20] ("stop bits (10: 1 bit)")
                n97 = call-poly "VISA Configure Serial Port"("VISA resource name"=w322, "timeout (10sec)"=u32 1000, "Enable Termination\nChar (T)"=FALSE ("Enable Termination\nChar (T)"), "baud rate (9600)"=u32 19200, "data bits (8)"=u16 8, "parity (0:none)"=enum16{"None", "Odd", "Even", "Mark", "Space"}."None", "error in (no error)"=w323, "stop bits (10: 1 bit)"=w328, "flow control (0:none)"=w329) -> ("VISA resource name out"=w320:refnum<visa-resource-name>, "error out"=w321:errorcluster)  [unwired: 5 in]
              }
            }
            n98 = disable-structure shown="Enabled" {
              disable-tunnel: w276 -> [w298 w312]
              disable-tunnel: [w297 w311] -> w272
              disable-tunnel: [w296 w310] -> w275
              disable-tunnel: w274 -> [w295 w310]
              frame #0 {
                n99 = disable-structure shown="Enabled" {
                  disable-tunnel: w295 -> [w301 w303]
                  disable-tunnel: [w300 w303] -> w294
                  disable-tunnel: [w299 u32 1 ("Bytes at Port")] -> w293
                  frame #0 {
                    n100 = property class="Instr"(reference=w301) -> (reference out=w300:refnum<visa-resource-name>, "Serial Settings:Number of Bytes at Serial Port"=w299:u32)  [unwired: 1 in, 1 out]
                  }
                  frame #1 {
                  }
                }
                n101 = case shown="1, Default" w293 {
                  tunnel: w298 -> [w305 w309]
                  tunnel: [w305 w308] -> w297
                  tunnel: [w304 w307] -> w296
                  tunnel: w294 -> [w304 w306]
                  frame #0 {
                  }
                  frame #1 {
                    n102 = VISA Clear(VISA resource name=w306, error in (no error)=w309) -> (VISA resource name out=w307:refnum<visa-resource-name>, error out=w308:errorcluster)
                  }
                }
              }
              frame #1 {
                n103 = VISA Flush I/O Buffer(VISA resource name=w310, error in (no error)=w312) -> (error out=w311:errorcluster)  [unwired: 1 in, 1 out]
              }
            }
            n104 = case shown="Error" w272 {
              selector: w272 -> [w281 w288]
              tunnel: w280 -> [w285 w292]
              tunnel: [w284 w291] -> w279
              tunnel: w275 -> [w283 _]
              tunnel: ["" ("State(s) in Front (\"\")") "Macro: Exit" ("State(s) in Front (\"\")")] -> w271
              tunnel: [w281 w286] -> w270
              frame #0 {
                n105 = Bundle By Name(cluster=w285, "ComPort"=w283) -> (w284:T6)
              }
              frame #1 {
                n106 = Bundle By Name(cluster=w292, "Error Out Flag"=TRUE) -> (w291:T6)
                n107 = Bundle By Name(cluster=w288, "status"=FALSE) -> (w286:errorcluster)
              }
            }
          }
        }
        n108 = call <vilib>:"Add State(s) to Queue__jki_lib_state_machine.vi"("State(s) in Front (\"\")"=w235, "State(s) in (\"\")"=w243) -> ("States Out"=w242:string)  [unwired: 13 in]
      }
      frame #18 {
        w340 = u8 225  # ACK
        w353 = u8 227  # ETX
        w356 = u8 226  # STX
        # "Found that if set to 100, can run repeatedly.  But decided this should be in calling code in case\ntime critical data is needed."
        n109 = Unbundle By Name(w348) -> ("ComPort"=w366:refnum<visa-resource-name>)
        n110 = call "HEWH_DSM_CMD.vi"("Command"="Command") -> ("CMD Array"=w358:u8[])  [unwired: 10 in]
        n111 = Array Size(array=w358) -> (size(s)=w364:i32)
        n112 = Array Size(array="Command Data") -> (size(s)=w362:i32)
        n113 = Compound Arithmetic op=ADD(7 ("x"), w364, w362) -> (w360:i32)
        n114 = To Unsigned Byte Integer(number=w360) -> (unsigned 8bit integer=w361:u8)
        n115 = Build Array (concatenate)("Destination Address", w361, "Source Address", w358, "Command Data") -> (w355:u8[])
        n116 = call "crc16-ccitt (x1021).vi"("unsigned byte array"=w355) -> ("CRC"=w354:u8[])  [unwired: 9 in, 1 out]
        n117 = Build Array (concatenate)(w356, w355, w354, w353) -> (w342:u8[])
        n118 = call "Delay mS.vi"("Error In"=w334, "milliseconds to wait"=u32 100 ("milliseconds to wait 2")) -> ("Error Out"=w333:errorcluster)  [unwired: 13 in]
        n119 = call "GEA2 Add ESC Char.vi"("Message"=w342) -> ("Message Out"=w341:u8[])  [unwired: 14 in]
        "Command" <- w341
        n120 = flat-sequence {
          tunnel: [w388] -> w349
          tunnel: w333 -> [_]
          frame #0 {
            n121 = Tick Count (ms)() -> (millisecond timer value=w388:u32)
          }
        }
        n122 = Bundle By Name(cluster=w348, "HEWH Command"="Command") -> (w347:T6)
        n123 = disable-structure shown="Enabled" {
          disable-tunnel: w366 -> [w374 w380]
          disable-tunnel: w333 -> [w373 w379]
          disable-tunnel: [w372 w378] -> w352
          disable-tunnel: [w371 w377] -> w336
          disable-tunnel: w341 -> [w369 w376]
          disable-tunnel: w349 -> [_ w375]
          frame #0 {
            n124 = Byte Array To String(unsigned byte array=w369) -> (string=w370:string)
            n125 = VISA Write(VISA resource name=w374, write buffer=w370, error in (no error)=w373) -> (VISA resource name out=w372:refnum<visa-resource-name>, error out=w371:errorcluster)  [unwired: 1 out]
          }
          frame #1 {
            n126 = for {
              tunnel: w380 -> [w387]
              tunnel: w379 -> [w386]
              tunnel: w376 -> [w385] mode=indexing
              tunnel: [w384] -> w378
              tunnel: [w382] -> w377
              tunnel: w375 -> [_]
              n127 = Build Array(w385) -> (w381:u8[])
              n128 = Byte Array To String(unsigned byte array=w381) -> (string=w383:string)
              n129 = VISA Write(VISA resource name=w387, write buffer=w383, error in (no error)=w386) -> (VISA resource name out=w384:refnum<visa-resource-name>, error out=w382:errorcluster)  [unwired: 1 out]
            }
          }
        }
        n130 = Array Size(array=w341) -> (size(s)=w344:i32)
        n131 = Increment(x=w344) -> (x+1=w345:i32)
        n132 = Build Array (concatenate)(w341, w340) -> (w339:u8[])
        n133 = To Unsigned Long Integer(number=w345) -> (unsigned 32bit integer=w343:u32)
        n134 = call "Delay mS.vi"("Error In"=w336, "milliseconds to wait"=u32 200) -> ("Error Out"=w335:errorcluster)  [unwired: 13 in]
        n135 = Byte Array To String(unsigned byte array=w339) -> (string=w350:string)
        n136 = VISA Read(VISA resource name=w352, byte count=w343, error in (no error)=w335) -> (read buffer=w351:string, error out=w337:errorcluster)  [unwired: 2 out]
        n137 = Equal?(x=w350, y=w351) -> (x = y?=w338:bool)
        "WriteOK" <- w338
        n138 = call <vilib>:"Add State(s) to Queue__jki_lib_state_machine.vi"("State(s) in (\"\")"=w368) -> ("States Out"=w367:string)  [unwired: 14 in]
        n139 = local write "WriteACK"(w338) -> ()
        "tStart" <- w349
      }
      frame #19 {
        # "Your code here.\n(You can make a copy of, or modify, this frame)"
        n140 = Unbundle By Name(w395) -> ("ComPort"=w394:refnum<visa-resource-name>)
        n141 = for {
          tunnel: w394 -> [w408]
          tunnel: "Random Data" -> [w404] mode=indexing
          tunnel: [w401] -> w393 mode=indexing
          shift-right: [w400] -> w391
          shift-left: w392 -> [w399]
          n142 = Build Array(w404) -> (w405:u8[])
          n143 = Byte Array To String(unsigned byte array=w405) -> (string=w402:string)
          n144 = VISA Write(VISA resource name=w408, write buffer=w402, error in (no error)=w399) -> (VISA resource name out=w407:refnum<visa-resource-name>, error out=w398:errorcluster)  [unwired: 1 out]
          n145 = VISA Read(VISA resource name=w407, byte count=u32 1, error in (no error)=w398) -> (read buffer=w403:string, error out=w400:errorcluster)  [unwired: 2 out]
          n146 = Equal?(x=w402, y=w403) -> (x = y?=w401:bool)
        }
        n147 = And Array Elements(Boolean array=w393) -> (logical AND=w389:bool)
        n148 = local write "WriteOK"(w389) -> ()
        n149 = call <vilib>:"Add State(s) to Queue__jki_lib_state_machine.vi"("State(s) in (\"\")"=w397) -> ("States Out"=w396:string)  [unwired: 14 in]
      }
      frame #20 {
        # "Template Separator\n(You can make a copy of, or modify, this frame)"
        n150 = call <vilib>:"Add State(s) to Queue__jki_lib_state_machine.vi"("State(s) in (\"\")"=w412) -> ("States Out"=w411:string)  [unwired: 14 in]
      }
      frame #21 {
        # "Your code here.\n(You can make a copy of, or modify, this frame)"
        n151 = case shown="True" TRUE {
          tunnel: w417 -> [_ w430]
          tunnel: [u8[] [] ("unsigned byte array") w428] -> w416
          tunnel: ["ReadData: ACK" ("State(s) in Front (\"\")") "Data: Parse" ("State(s) in Front (\"\")")] -> w414
          tunnel: [_ w425] -> w413
          frame #0 {
          }
          frame #1 {
            n152 = Unbundle By Name(w430) -> ("ComPort"=w427:refnum<visa-resource-name>)
            n153 = call "GEA2 Check Read Ready.vi"("reference"=w427) -> ("Bytes at Port"=w425:u32)  [unwired: 10 in]
            "byte count" <- w425
            n154 = VISA Read(VISA resource name=w427, byte count=w425) -> (read buffer=w429:string)  [unwired: 1 in, 3 out]
            n155 = String To Byte Array(string=w429) -> (unsigned byte array=w428:u8[])
            n156 = local write "ReadArray"(w428) -> ()
          }
        }
        n157 = Bundle By Name(cluster=w417, "Total Bytes Read"=w413, "ReadArray"=w416, "CRCArray"=u8[] [] ("ReadArray")) -> (w419:T6)
        n158 = call <vilib>:"Add State(s) to Queue__jki_lib_state_machine.vi"("State(s) in Front (\"\")"=w414, "State(s) in (\"\")"=w422) -> ("States Out"=w421:string)  [unwired: 13 in]
      }
      frame #22 {
        w435 = u8 225  # ACK
        # "Read ACK Byte"
        n159 = Unbundle By Name(w447) -> ("ComPort"=w433:refnum<visa-resource-name>, "ReadArray"=w434:u8[], "HEWH Command"=w431:u8)
        n160 = local write "ReadArray"(w434) -> ()
        n161 = VISA Read(VISA resource name=w433, byte count=u32 1, error in (no error)=w440) -> (read buffer=w444:string, error out=w438:errorcluster)  [unwired: 2 out]
        n162 = property class="Instr"(reference=w433) -> ("Serial Settings:Number of Bytes at Serial Port"=→"Serial Settings:Number of Bytes at Serial Port 2":u32)  [unwired: 1 in, 2 out]
        n163 = String To Byte Array(string=w444) -> (unsigned byte array=w443:u8[])
        n164 = Index Array(array=w443, index=0) -> (element=w441:u8)
        n165 = Build Array (concatenate)(w434, w443) -> (w448:u8[])
        n166 = Equal?(x=w441, y=w435) -> (x = y?=w439:bool)
        "WriteACK" <- w439
        n167 = Bundle By Name(cluster=w447, "ReadArray"=w448) -> (w446:T6)
        n168 = case shown="False" w439 {
          tunnel: w438 -> [w453 w458]
          tunnel: [w451 w458] -> w437
          tunnel: ["ReadData: Rest" ("State(s) in Front (\"\")") w457] -> w436
          tunnel: w431 -> [_ w456]
          frame #0 {
            n169 = call "Error Bool Enumerator.vi"("Error Enum"=HEWH_Error_Enumeration."GEA2 ReadACK", "Error In"=w453) -> ("Error Out"=w451:errorcluster)  [unwired: 7 in]
          }
          frame #1 {
            n170 = call "HEWH Command Needs Read.vi"("Command"=w456) -> ("RQST"=w455:bool)  [unwired: 13 in, 1 out]
            n171 = case shown="False" w455 {
              tunnel: ["ReadData: STX" ("State(s) in Front (\"\")") "Macro: Exit" ("State(s) in Front (\"\")")] -> w457
              frame #0 {
              }
              frame #1 {
              }
            }
          }
        }
        n172 = call <vilib>:"Add State(s) to Queue__jki_lib_state_machine.vi"("State(s) in Front (\"\")"=w436, "State(s) in (\"\")"=w450) -> ("States Out"=w449:string)  [unwired: 13 in]
      }
      frame #23 {
        w470 = u8 224  # ESC
        # "Read Destination byte.  If its your message, than continue to length, otherwise, read the rest of the message."
        n173 = Unbundle By Name(w483) -> ("ComPort"=w463:refnum<visa-resource-name>, "ReadArray"=w461:u8[])
        n174 = VISA Read(VISA resource name=w463, byte count=u32 1, error in (no error)=w477) -> (read buffer=w480:string, error out=w465:errorcluster)  [unwired: 2 out]
        n175 = String To Byte Array(string=w480) -> (unsigned byte array=w467:u8[])
        n176 = Index Array(array=w467, index=0) -> (element=w472:u8)
        n177 = local write "ReadArray"(w461) -> ()
        n178 = Equal?(x=w472, y=w470) -> (x = y?=w469:bool)
        n179 = case shown="True" w469 {
          tunnel: [w488 w489] -> w468
          tunnel: w467 -> [w488 w496]
          tunnel: [w487 w490] -> w466
          tunnel: w461 -> [w487 w497]
          tunnel: w465 -> [w486 w493]
          tunnel: [w486 w492] -> w464
          tunnel: w463 -> [_ w491]
          frame #0 {
          }
          frame #1 {
            n180 = VISA Read(VISA resource name=w491, byte count=u32 1, error in (no error)=w493) -> (read buffer=w495:string, error out=w492:errorcluster)  [unwired: 2 out]
            n181 = String To Byte Array(string=w495) -> (unsigned byte array=w489:u8[])
            n182 = Build Array (concatenate)(w497, w496) -> (w490:u8[])
          }
        }
        n183 = Build Array (concatenate)(w466, w468) -> (w462:u8[])
        n184 = local read "Source Address"() -> (w473:u8)
        n185 = Index Array(array=w468, index=0) -> (element=w478:u8)
        n186 = Bundle By Name(cluster=w483, "ReadArray"=w462, "CRCArray"=w468) -> (w482:T6)
        n187 = Equal?(x=w478, y=w473) -> (x = y?=w476:bool)
        n188 = case shown="False" w476 {
          tunnel: w464 -> [w501 w503]
          tunnel: [w499 w503] -> w475
          tunnel: ["ReadData: Rest" ("State(s) in Front (\"\")") "ReadData: Length" ("State(s) in Front (\"\")")] -> w474
          frame #0 {
            n189 = call <vilib>:"Merge Errors.vi"("error in 2 (no error)"=errorcluster {"status"=FALSE, "code"=7000, "source"="Message not for Me"}, "error in 1 (no error)"=w501) -> ("error out"=w499:errorcluster)  [unwired: 5 in]
          }
          frame #1 {
          }
        }
        n190 = call <vilib>:"Add State(s) to Queue__jki_lib_state_machine.vi"("State(s) in Front (\"\")"=w474, "State(s) in (\"\")"=w485) -> ("States Out"=w484:string)  [unwired: 13 in]
      }
      frame #24 {
        w518 = u8 224  # ESC
        # "Your code here.\n(You can make a copy of, or modify, this frame)"
        n191 = Unbundle By Name(w529) -> ("ComPort"=w512:refnum<visa-resource-name>, "ReadArray"=w510:u8[], "CRCArray"=w504:u8[])
        n192 = VISA Read(VISA resource name=w512, byte count=u32 1, error in (no error)=w524) -> (read buffer=w526:string, error out=w514:errorcluster)  [unwired: 2 out]
        n193 = String To Byte Array(string=w526) -> (unsigned byte array=w516:u8[])
        n194 = local write "ReadArray"(w510) -> ()
        n195 = Index Array(array=w516, index=0) -> (element=w520:u8)
        n196 = Equal?(x=w520, y=w518) -> (x = y?=w517:bool)
        n197 = case shown="True" w517 {
          tunnel: [w535 w536] -> w505
          tunnel: w516 -> [w535 w543]
          tunnel: [w534 w537] -> w515
          tunnel: w510 -> [w534 w544]
          tunnel: w514 -> [w533 w540]
          tunnel: [w533 w539] -> w513
          tunnel: w512 -> [_ w538]
          frame #0 {
          }
          frame #1 {
            n198 = VISA Read(VISA resource name=w538, byte count=u32 1, error in (no error)=w540) -> (read buffer=w542:string, error out=w539:errorcluster)  [unwired: 2 out]
            n199 = String To Byte Array(string=w542) -> (unsigned byte array=w536:u8[])
            n200 = Build Array (concatenate)(w544, w543) -> (w537:u8[])
          }
        }
        n201 = Index Array(array=w505, index=0) -> (element=w509:u8)
        n202 = Build Array (concatenate)(w515, w505) -> (w530:u8[])
        n203 = Subtract(x=w509, y=u8 6) -> (x-y=w507:u8)
        n204 = Build Array (concatenate)(w504, w505) -> (w506:u8[])
        n205 = Less Or Equal?(x=w507, y=u8 0 ("0")) -> (x <= y?=w523:bool)
        n206 = Bundle By Name(cluster=w529, "ReadArray"=w530, "CRCArray"=w506, "Bytes Remaining"=w507) -> (w528:T6)
        n207 = case shown="False" w523 {
          tunnel: w513 -> [w546 w550]
          tunnel: [w546 w548] -> w522
          tunnel: ["ReadData: Bytes" ("State(s) in Front (\"\")") "ReadData: Rest" ("State(s) in Front (\"\")")] -> w521
          frame #0 {
          }
          frame #1 {
            n208 = call <vilib>:"Merge Errors.vi"("error in 2 (no error)"=errorcluster {"status"=FALSE, "code"=7000, "source"="0 Length"}, "error in 1 (no error)"=w550) -> ("error out"=w548:errorcluster)  [unwired: 5 in]
          }
        }
        n209 = call <vilib>:"Add State(s) to Queue__jki_lib_state_machine.vi"("State(s) in Front (\"\")"=w521, "State(s) in (\"\")"=w532) -> ("States Out"=w531:string)  [unwired: 13 in]
      }
      frame #25 {
        w564 = u8 224  # ESC
        # "Your code here.\n(You can make a copy of, or modify, this frame)"
        n210 = Unbundle By Name(w573) -> ("ComPort"=w558:refnum<visa-resource-name>, "ReadArray"=w554:u8[], "Bytes Remaining"=w556:u8, "CRCArray"=w551:u8[])
        n211 = VISA Read(VISA resource name=w558, byte count=u32 1, error in (no error)=w569) -> (read buffer=w570:string, error out=w560:errorcluster)  [unwired: 2 out]
        n212 = String To Byte Array(string=w570) -> (unsigned byte array=w562:u8[])
        n213 = Index Array(array=w562, index=0) -> (element=w566:u8)
        n214 = Equal?(x=w566, y=w564) -> (x = y?=w563:bool)
        n215 = case shown="True" w563 {
          tunnel: [w579 w580] -> w553
          tunnel: w562 -> [w579 w587]
          tunnel: [w578 w581] -> w561
          tunnel: w554 -> [w578 w588]
          tunnel: w560 -> [w577 w584]
          tunnel: [w577 w583] -> w559
          tunnel: w558 -> [_ w582]
          frame #0 {
          }
          frame #1 {
            n216 = VISA Read(VISA resource name=w582, byte count=u32 1, error in (no error)=w584) -> (read buffer=w586:string, error out=w583:errorcluster)  [unwired: 2 out]
            n217 = String To Byte Array(string=w586) -> (unsigned byte array=w580:u8[])
            n218 = Build Array (concatenate)(w588, w587) -> (w581:u8[])
          }
        }
        n219 = local write "ReadArray"(w554) -> ()
        n220 = Decrement(x=w556) -> (x-1=w555:u8)
        n221 = Build Array (concatenate)(w551, w553) -> (w552:u8[])
        n222 = Build Array (concatenate)(w561, w553) -> (w574:u8[])
        n223 = Greater Than 0?(x=w555) -> (x > 0?=w557:bool)
        n224 = Bundle By Name(cluster=w573, "ReadArray"=w574, "CRCArray"=w552, "Bytes Remaining"=w555) -> (w572:T6)
        n225 = case shown="False" w557 {
          tunnel: w559 -> [w592 w594]
          tunnel: [w590 w594] -> w568
          tunnel: ["ReadData: CRC1" ("State(s) in Front (\"\")") "ReadData: Bytes" ("State(s) in Front (\"\")")] -> w567
          frame #0 {
            n226 = call <vilib>:"Merge Errors.vi"("error in 2 (no error)"=errorcluster {"status"=FALSE, "code"=7000, "source"="0 Length"}, "error in 1 (no error)"=w592) -> ("error out"=w590:errorcluster)  [unwired: 5 in]
          }
          frame #1 {
          }
        }
        n227 = call <vilib>:"Add State(s) to Queue__jki_lib_state_machine.vi"("State(s) in Front (\"\")"=w567, "State(s) in (\"\")"=w576) -> ("States Out"=w575:string)  [unwired: 13 in]
      }
      frame #26 {
        w603 = u8 224  # ESC
        # "Your code here.\n(You can make a copy of, or modify, this frame)"
        n228 = Unbundle By Name(w611) -> ("ComPort"=w597:refnum<visa-resource-name>, "ReadArray"=w599:u8[])
        n229 = VISA Read(VISA resource name=w597, byte count=u32 1, error in (no error)=w607) -> (read buffer=w608:string, error out=w598:errorcluster)  [unwired: 2 out]
        n230 = String To Byte Array(string=w608) -> (unsigned byte array=w601:u8[])
        n231 = Index Array(array=w601, index=0) -> (element=w605:u8)
        n232 = Equal?(x=w605, y=w603) -> (x = y?=w602:bool)
        n233 = case shown="True" w602 {
          tunnel: [w617 w618] -> w596
          tunnel: w601 -> [w617 w625]
          tunnel: [w616 w619] -> w600
          tunnel: w599 -> [w616 w626]
          tunnel: w598 -> [w615 w622]
          tunnel: [w615 w621] -> w595
          tunnel: w597 -> [_ w620]
          frame #0 {
          }
          frame #1 {
            n234 = VISA Read(VISA resource name=w620, byte count=u32 1, error in (no error)=w622) -> (read buffer=w624:string, error out=w621:errorcluster)  [unwired: 2 out]
            n235 = String To Byte Array(string=w624) -> (unsigned byte array=w618:u8[])
            n236 = Build Array (concatenate)(w626, w625) -> (w619:u8[])
          }
        }
        n237 = Build Array (concatenate)(w600, w596) -> (w612:u8[])
        n238 = Bundle By Name(cluster=w611, "ReadArray"=w612, "CRCRead"=w596) -> (w610:T6)
        n239 = call <vilib>:"Add State(s) to Queue__jki_lib_state_machine.vi"("State(s) in Front (\"\")"="ReadData: CRC2" ("State(s) in Front (\"\")"), "State(s) in (\"\")"=w614) -> ("States Out"=w613:string)  [unwired: 13 in]
      }
      frame #27 {
        w638 = u8 224  # ESC
        # "Your code here.\n(You can make a copy of, or modify, this frame)"
        n240 = Unbundle By Name(w646) -> ("ComPort"=w633:refnum<visa-resource-name>, "ReadArray"=w629:u8[], "CRCRead"=w628:u8[])
        n241 = VISA Read(VISA resource name=w633, byte count=u32 1, error in (no error)=w642) -> (read buffer=w643:string, error out=w634:errorcluster)  [unwired: 2 out]
        n242 = String To Byte Array(string=w643) -> (unsigned byte array=w636:u8[])
        n243 = Index Array(array=w636, index=0) -> (element=w640:u8)
        n244 = Equal?(x=w640, y=w638) -> (x = y?=w637:bool)
        n245 = case shown="True" w637 {
          tunnel: [w651 w652] -> w630
          tunnel: w636 -> [w651 w659]
          tunnel: [w650 w653] -> w635
          tunnel: w629 -> [w650 w660]
          tunnel: w634 -> [w649 w656]
          tunnel: [w649 w655] -> w632
          tunnel: w633 -> [_ w654]
          frame #0 {
          }
          frame #1 {
            n246 = VISA Read(VISA resource name=w654, byte count=u32 1, error in (no error)=w656) -> (read buffer=w658:string, error out=w655:errorcluster)  [unwired: 2 out]
            n247 = String To Byte Array(string=w658) -> (unsigned byte array=w652:u8[])
            n248 = Build Array (concatenate)(w660, w659) -> (w653:u8[])
          }
        }
        n249 = local write "ReadArray"(w629) -> ()
        n250 = Build Array (concatenate)(w635, w630) -> (w631:u8[])
        n251 = Build Array (concatenate)(w628, w630) -> (w627:u8[])
        n252 = Bundle By Name(cluster=w646, "ReadArray"=w631, "CRCRead"=w627) -> (w645:T6)
        n253 = local write "CRCRead"(w627) -> ()
        n254 = call <vilib>:"Add State(s) to Queue__jki_lib_state_machine.vi"("State(s) in Front (\"\")"="ReadData: CheckCRC" ("State(s) in Front (\"\")"), "State(s) in (\"\")"=w648) -> ("States Out"=w647:string)  [unwired: 13 in]
      }
      frame #28 {
        # "Your code here.\n(You can make a copy of, or modify, this frame)"
        n255 = Unbundle By Name(w663) -> ("CRCRead"=w668:u8[], "CRCArray"=w665:u8[])
        "DataReturned" <- w665
        n256 = call "crc16-ccitt (x1021).vi"("error in (no error)"=w669, "unsigned byte array"=w665) -> ("error out (dup)"=w666:errorcluster, "CRC"=w664:u8[])  [unwired: 8 in]
        n257 = Equal?(x=w668, y=w664) -> (x = y?=w661:bool)
        "CRC Match" <- w661
        n258 = case shown="True" w661 {
          tunnel: ["ReadData: Rest" ("State(s) in Front (\"\")") "ReadData: ETX" ("State(s) in Front (\"\")")] -> w670
          tunnel: [w676 w678] -> w667
          tunnel: w666 -> [w675 w678]
          frame #0 {
            n259 = call "Error Bool Enumerator.vi"("Error Enum"=HEWH_Error_Enumeration."GEA2 CRC Mismatch", "Error In"=w675, "Error?"=TRUE) -> ("Error Out"=w676:errorcluster)  [unwired: 6 in]
          }
          frame #1 {
          }
        }
        n260 = Bundle By Name(cluster=w663, "CRC"=w661) -> (w662:T6)
        n261 = call <vilib>:"Add State(s) to Queue__jki_lib_state_machine.vi"("State(s) in Front (\"\")"=w670, "State(s) in (\"\")"=w672) -> ("States Out"=w671:string)  [unwired: 13 in]
      }
      frame #29 {
        w683 = u8 226  # STX
        # "Your code here.\n(You can make a copy of, or modify, this frame)"
        n262 = Unbundle By Name(w695) -> ("ComPort"=w681:refnum<visa-resource-name>, "ReadArray"=w697:u8[])
        n263 = VISA Read(VISA resource name=w681, byte count=u32 1, error in (no error)=w693) -> (VISA resource name out=w680:refnum<visa-resource-name>, read buffer=w687:string, error out=w691:errorcluster)  [unwired: 1 out]
        n264 = String To Byte Array(string=w687) -> (unsigned byte array=w686:u8[])
        n265 = property class="Instr"(reference=w680) -> ("Serial Settings:Number of Bytes at Serial Port"=→"Serial Settings:Number of Bytes at Serial Port 3":u32)  [unwired: 1 in, 2 out]
        n266 = Index Array(array=w686, index=0) -> (element=w684:u8)
        n267 = Build Array (concatenate)(w697, w686) -> (w696:u8[])
        n268 = Equal?(x=w684, y=w683) -> (x = y?=w692:bool)
        n269 = case shown="False" w692 {
          tunnel: w691 -> [w703 w706]
          tunnel: [w700 w706] -> w690
          tunnel: ["ReadData: Rest" ("State(s) in Front (\"\")") "ReadData: Destination" ("State(s) in Front (\"\")")] -> w689
          frame #0 {
            n270 = call "Error Bool Enumerator.vi"("Error Enum"=HEWH_Error_Enumeration."GEA2 STX", "Error In"=w703, "Error?"=TRUE) -> ("Error Out"=w700:errorcluster)  [unwired: 6 in]
          }
          frame #1 {
          }
        }
        n271 = Bundle By Name(cluster=w695, "ReadArray"=w696) -> (w694:T6)
        n272 = call <vilib>:"Add State(s) to Queue__jki_lib_state_machine.vi"("State(s) in Front (\"\")"=w689, "State(s) in (\"\")"=w699) -> ("States Out"=w698:string)  [unwired: 13 in]
      }
      frame #30 {
        w707 = u8 227  # ETX
        # "Your code here.\n(You can make a copy of, or modify, this frame)"
        n273 = Unbundle By Name(w719) -> ("ComPort"=w722:refnum<visa-resource-name>, "ReadArray"=w721:u8[])
        n274 = VISA Read(VISA resource name=w722, byte count=u32 1, error in (no error)=w717) -> (read buffer=w711:string, error out=w715:errorcluster)  [unwired: 2 out]
        n275 = String To Byte Array(string=w711) -> (unsigned byte array=w710:u8[])
        n276 = Index Array(array=w710, index=0) -> (element=w708:u8)
        n277 = Build Array (concatenate)(w721, w710) -> (w720:u8[])
        n278 = Equal?(x=w708, y=w707) -> (x = y?=w716:bool)
        n279 = Bundle By Name(cluster=w719, "ReadArray"=w720) -> (w718:T6)
        n280 = case shown="True" w716 {
          tunnel: w715 -> [w727 w731]
          tunnel: [w729 w731] -> w714
          tunnel: ["ReadData: Rest" ("State(s) in Front (\"\")") "ReadData: SendACK" ("State(s) in Front (\"\")")] -> w713
          frame #0 {
            n281 = call "Error Bool Enumerator.vi"("Error Enum"=HEWH_Error_Enumeration."GEA2 ETX", "Error In"=w727, "Error?"=TRUE) -> ("Error Out"=w729:errorcluster)  [unwired: 6 in]
          }
          frame #1 {
          }
        }
        n282 = call <vilib>:"Add State(s) to Queue__jki_lib_state_machine.vi"("State(s) in Front (\"\")"=w713, "State(s) in (\"\")"=w724) -> ("States Out"=w723:string)  [unwired: 13 in]
      }
      frame #31 {
        n283 = Unbundle By Name(w742) -> ("ComPort"=w739:refnum<visa-resource-name>, "ReadArray"=w743:u8[])
        n284 = disable-structure shown="Enabled" {
          disable-tunnel: w739 -> [w748 w750]
          disable-tunnel: [w747 w750] -> w738
          disable-tunnel: [w746 u32 100 ("Bytes at Port")] -> w735
          frame #0 {
            n285 = property class="Instr"(reference=w748) -> (reference out=w747:refnum<visa-resource-name>, "Serial Settings:Number of Bytes at Serial Port"=w746:u32)  [unwired: 1 in, 1 out]
          }
          frame #1 {
          }
        }
        n286 = VISA Read(VISA resource name=w738, byte count=w735) -> (read buffer=w737:string, error out=w732:errorcluster)  [unwired: 1 in, 2 out]
        "error out" <- w732
        n287 = String To Byte Array(string=w737) -> (unsigned byte array=w736:u8[])
        n288 = Build Array (concatenate)(w743, w736) -> (w740:u8[])
        n289 = local write "ReadArray"(w740) -> ()
        n290 = Bundle By Name(cluster=w742, "ReadArray"=w740) -> (w741:T6)
        n291 = call <vilib>:"Merge Errors.vi"("error in 2 (no error)"=w733, "error in 1 (no error)"=w732) -> ("error out"=w734:errorcluster)  [unwired: 5 in]
        n292 = call <vilib>:"Add State(s) to Queue__jki_lib_state_machine.vi"("State(s) in (\"\")"=w745) -> ("States Out"=w744:string)  [unwired: 14 in]
      }
      frame #32 {
        w765 = u8 225  # ACK
        n293 = Unbundle By Name(w753) -> ("ReadArray"=w755:u8[], "ComPort"=w758:refnum<visa-resource-name>)
        n294 = property class="Instr"(reference=w758) -> ("Serial Settings:Number of Bytes at Serial Port"=→"Serial Settings:Number of Bytes at Serial Port":u32)  [unwired: 1 in, 2 out]
        n295 = Build Array(w765) -> (w768:u8[])
        n296 = Byte Array To String(unsigned byte array=w768) -> (string=w767:string)
        n297 = VISA Write(VISA resource name=w758, write buffer=w767, error in (no error)=w771) -> (VISA resource name out=w770:refnum<visa-resource-name>, error out=w766:errorcluster)  [unwired: 1 out]
        n298 = VISA Read(VISA resource name=w770, byte count=u32 1, error in (no error)=w766) -> (read buffer=w763:string, error out=w764:errorcluster)  [unwired: 2 out]
        n299 = Equal?(x=w767, y=w763) -> (x = y?=w761:bool)
        "Read_ACK" <- w761
        n300 = String To Byte Array(string=w763) -> (unsigned byte array=w754:u8[])
        "ACK(E1?)" <- w754
        n301 = Not(x=w761) -> (.not. x?=w760:bool)
        n302 = Build Array (concatenate)(w755, w754) -> (w751:u8[])
        n303 = local write "ReadArray"(w751) -> ()
        n304 = call "Error Bool Enumerator.vi"("Error Enum"=HEWH_Error_Enumeration."GEA2 Send ACK Mismatch", "Error In"=w764, "Error?"=w760) -> ("Error Out"=w756:errorcluster)  [unwired: 6 in]
        n305 = Bundle By Name(cluster=w753, "ReadArray"=w751) -> (w752:T6)
        n306 = case shown="No Error" w756 {
          tunnel: ["Macro: Exit" ("State(s) in Front (\"\")") "ReadData: Rest" ("State(s) in Front (\"\")")] -> w759
          frame #0 {
          }
          frame #1 {
          }
        }
        n307 = call <vilib>:"Add State(s) to Queue__jki_lib_state_machine.vi"("State(s) in Front (\"\")"=w759, "State(s) in (\"\")"=w773) -> ("States Out"=w772:string)  [unwired: 13 in]
      }
      frame #33 {
        # "Template Separator\n(You can make a copy of, or modify, this frame)"
        n308 = call <vilib>:"Add State(s) to Queue__jki_lib_state_machine.vi"("State(s) in (\"\")"=w779) -> ("States Out"=w778:string)  [unwired: 14 in]
      }
      frame #34 {
        # "Template Separator\n(You can make a copy of, or modify, this frame)"
        n309 = Unbundle By Name(w783) -> ("Total Bytes Read"=w784:u32)
        n310 = To Long Integer(number=w784) -> (32bit integer=w782:i32)
        n311 = Equal To 0?(x=w782) -> (x = 0?=w781:bool)
        n312 = case shown="False" w781 {
          tunnel: [_ "Parse: STX\nParse: Destination\nParse: Length\nParse: Source\nParse: Bytes Data\nParse: CRC1\nParse: CRC2\nCheckCRC\nParse: ETX" ("State(s) in Front (\"\")")] -> w780
          tunnel: w783 -> [w791 w792]
          tunnel: [w790 w792] -> w785
          frame #0 {
            n313 = Bundle By Name(cluster=w791, "Bytes Data"=u8[] []) -> (w790:T6)
          }
          frame #1 {
            # "Note, check complete left out.  If there is more\nthan one message, the balance is discarded."
          }
        }
        n314 = call <vilib>:"Add State(s) to Queue__jki_lib_state_machine.vi"("State(s) in Front (\"\")"=w780, "State(s) in (\"\")"=w788) -> ("States Out"=w787:string)  [unwired: 13 in]
      }
      frame #35 {
        # "Template Separator\n(You can make a copy of, or modify, this frame)"
        n315 = Unbundle By Name(w795) -> ("Total Bytes Read"=w803:u32, "Current Read Index"=w802:i32, "ReadArray"=w800:u8[])
        "Current Read Index" <- w802
        n316 = while {
          tunnel: [w812] -> w799
          tunnel: w803 -> [w811]
          shift-right: [w808] -> w804
          shift-left: w802 -> [w809]
          tunnel: w800 -> [w815]
          stop <- w813 stop-if-true
          w807 = u8 226  # STX
          n317 = Increment(x=w809) -> (x+1=w808:i32)
          n318 = Index Array(array=w815, index=w809) -> (element=w814:u8)
          n319 = Less?(x=w811, y=w808) -> (x < y?=w810:bool)
          n320 = Equal?(x=w814, y=w807) -> (x = y?=w812:bool)
          n321 = Or(x=w810, y=w812) -> (x .or. y?=w813:bool)
        }
        n322 = case shown="False" w799 {
          tunnel: w798 -> [w819 w827]
          tunnel: [w817 w827] -> w797
          tunnel: ["Exit" ("State(s) in Front (\"\")") _] -> w796
          frame #0 {
            n323 = disable-structure shown="Enabled" {
              disable-tunnel: w819 -> [w822 w826]
              disable-tunnel: [w820 w826] -> _
              disable-tunnel: [_ w825] -> w817
              frame #0 {
                n324 = call "Error Bool Enumerator.vi"("Error Enum"=HEWH_Error_Enumeration."GEA2 STX", "Error In"=w822, "Error?"=TRUE) -> ("Error Out"=w820:errorcluster)  [unwired: 6 in]
              }
              frame #1 {
                # "Partial Message"
                n325 = Bundle By Name(cluster=w826, "source"="Partial GEA Message") -> (w825:errorcluster)
              }
            }
            n326 = local write "Partial Message"(TRUE ("Partial Message")) -> ()
          }
          frame #1 {
          }
        }
        n327 = Bundle By Name(cluster=w795, "Current Read Index"=w804, "Bytes Data"=u8[] []) -> (w794:T6)
        n328 = call <vilib>:"Add State(s) to Queue__jki_lib_state_machine.vi"("State(s) in Front (\"\")"=w796, "State(s) in (\"\")"=w806) -> ("States Out"=w805:string)  [unwired: 13 in]
      }
      frame #36 {
        w830 = u8 224  # ESC
        # "Template Separator\n(You can make a copy of, or modify, this frame)"
        n329 = Unbundle By Name(w829) -> ("CRCArray"=w832:u8[], "ReadArray"=w836:u8[], "Current Read Index"=w834:i32)  [unwired: 1 out]
        n330 = Increment(x=w834) -> (x+1=w837:i32)
        n331 = Index Array(array=w836, index=w834) -> (element=w835:u8)
        n332 = Equal?(x=w835, y=w830) -> (x = y?=w831:bool)
        n333 = case shown="True" w831 {
          tunnel: [w844 w847] -> w839
          tunnel: [w843 w845] -> w838
          tunnel: w836 -> [_ w848]
          tunnel: w835 -> [w844 _]
          tunnel: w837 -> [w843 w846]
          frame #0 {
          }
          frame #1 {
            n334 = Increment(x=w846) -> (x+1=w845:i32)
            n335 = Index Array(array=w848, index=w846) -> (element=w847:u8)
          }
        }
        "Source Read" <- w839
        n336 = Build Array (concatenate)(w832, w839) -> (w833:u8[])
        n337 = Bundle By Name(cluster=w829, "CRCArray"=w833, "Current Read Index"=w838) -> (w828:T6)
        n338 = call <vilib>:"Add State(s) to Queue__jki_lib_state_machine.vi"("State(s) in (\"\")"=w842) -> ("States Out"=w841:string)  [unwired: 14 in]
      }
      frame #37 {
        w856 = -3  # CRC + ETX
        w852 = u8 224  # ESC
        # "Template Separator\n(You can make a copy of, or modify, this frame)"
        n339 = Unbundle By Name(w851) -> ("Total Bytes Read"=w862:u32, "ReadArray"=w858:u8[], "CRCArray"=w855:u8[], "Current Read Index"=w859:i32)  [unwired: 1 out]
        n340 = Increment(x=w859) -> (x+1=w860:i32)
        n341 = Index Array(array=w858, index=w859) -> (element=w861:u8)
        n342 = Equal?(x=w861, y=w852) -> (x = y?=w853:bool)
        n343 = case shown="False" w853 {
          tunnel: [w870 w872] -> w865
          tunnel: [w871 w873] -> w864
          tunnel: w858 -> [_ w875]
          tunnel: w860 -> [w871 w874]
          tunnel: w861 -> [w870 _]
          frame #0 {
          }
          frame #1 {
            n344 = Index Array(array=w875, index=w874) -> (element=w872:u8)
            n345 = Increment(x=w874) -> (x+1=w873:i32)
          }
        }
        "Length" <- w865
        n346 = Build Array (concatenate)(w855, w865) -> (w854:u8[])
        n347 = To Long Integer(number=w865) -> (32bit integer=w866:i32)
        n348 = Bundle By Name(cluster=w851, "Current Read Index"=w864, "CRCArray"=w854, "Bytes Remaining"=w865) -> (w850:T6)
        n349 = Compound Arithmetic op=ADD(w864, w856, w866) -> (w857:i32)
        n350 = To Long Integer(number=w857) -> (32bit integer=w863:i32)
        n351 = Less?(x=w862, y=w863) -> (x < y?=w849:bool)
        n352 = local write "Partial Message"(w849) -> ()
        n353 = call <vilib>:"Add State(s) to Queue__jki_lib_state_machine.vi"("State(s) in (\"\")"=w869) -> ("States Out"=w868:string)  [unwired: 14 in]
      }
      frame #38 {
        w878 = u8 224  # ESC
        # "Template Separator\n(You can make a copy of, or modify, this frame)"
        n354 = Unbundle By Name(w877) -> ("ReadArray"=w886:u8[], "Current Read Index"=w881:i32)
        n355 = Increment(x=w881) -> (x+1=w882:i32)
        n356 = Index Array(array=w886, index=w881) -> (element=w885:u8)
        n357 = Equal?(x=w885, y=w878) -> (x = y?=w879:bool)
        n358 = case shown="True" w879 {
          tunnel: [w891 w892] -> w883
          tunnel: [w890 w894] -> w880
          tunnel: w886 -> [_ w895]
          tunnel: w882 -> [w890 w893]
          tunnel: w885 -> [w891 _]
          frame #0 {
          }
          frame #1 {
            n359 = Index Array(array=w895, index=w893) -> (element=w892:u8)
            n360 = Increment(x=w893) -> (x+1=w894:i32)
          }
        }
        "Destination Read" <- w883
        n361 = Build Array(w883) -> (w884:u8[])
        n362 = Bundle By Name(cluster=w877, "Current Read Index"=w880, "CRCArray"=w884) -> (w876:T6)
        n363 = call <vilib>:"Add State(s) to Queue__jki_lib_state_machine.vi"("State(s) in (\"\")"=w889) -> ("States Out"=w888:string)  [unwired: 14 in]
      }
      frame #39 {
        w901 = u8 224  # ESC
        # "Template Separator\n(You can make a copy of, or modify, this frame)"
        n364 = Unbundle By Name(w900) -> ("ReadArray"=w913:u8[], "CRCArray"=w904:u8[], "Bytes Remaining"=w905:u8, "Bytes Data"=w907:u8[], "Current Read Index"=w914:i32)
        n365 = Increment(x=w914) -> (x+1=w915:i32)
        n366 = Index Array(array=w913, index=w914) -> (element=w916:u8)
        n367 = Equal?(x=w916, y=w901) -> (x = y?=w902:bool)
        n368 = case shown="True" w902 {
          tunnel: [w920 w922] -> w909
          tunnel: [w921 w925] -> w906
          tunnel: w913 -> [_ w924]
          tunnel: w913 -> [_ _]
          tunnel: w915 -> [w921 w923]
          tunnel: w916 -> [w920 _]
          frame #0 {
          }
          frame #1 {
            n369 = Index Array(array=w924, index=w923) -> (element=w922:u8)
            n370 = Increment(x=w923) -> (x+1=w925:i32)
          }
        }
        n371 = Decrement(x=w905) -> (x-1=w910:u8)
        n372 = Build Array (concatenate)(w907, w909) -> (w908:u8[])
        n373 = Build Array (concatenate)(w904, w909) -> (w903:u8[])
        n374 = Subtract(x=w910, y=u8 7) -> (x-y=w912:u8)
        n375 = Bundle By Name(cluster=w900, "Current Read Index"=w906, "CRCArray"=w903, "Bytes Remaining"=w910, "Bytes Data"=w908) -> (w899:T6)
        n376 = Greater Than 0?(x=w912) -> (x > 0?=w897:bool)
        n377 = case shown="True" w897 {
          tunnel: [_ "Parse: Bytes Data" ("State(s) in Front (\"\")")] -> w896
          frame #0 {
          }
          frame #1 {
          }
        }
        n378 = call <vilib>:"Add State(s) to Queue__jki_lib_state_machine.vi"("State(s) in Front (\"\")"=w896, "State(s) in (\"\")"=w918) -> ("States Out"=w917:string)  [unwired: 13 in]
      }
      frame #40 {
        w928 = u8 224  # ESC
        # "Template Separator\n(You can make a copy of, or modify, this frame)"
        n379 = Unbundle By Name(w927) -> ("ReadArray"=w932:u8[], "Current Read Index"=w933:i32)  [unwired: 1 out]
        n380 = Increment(x=w933) -> (x+1=w934:i32)
        n381 = Index Array(array=w932, index=w933) -> (element=w935:u8)
        n382 = Equal?(x=w935, y=w928) -> (x = y?=w929:bool)
        n383 = case shown="False" w929 {
          tunnel: [w940 w942] -> w931
          tunnel: [w941 w945] -> w930
          tunnel: w932 -> [_ w944]
          tunnel: w934 -> [w941 w943]
          tunnel: w935 -> [w940 _]
          frame #0 {
          }
          frame #1 {
            n384 = Index Array(array=w944, index=w943) -> (element=w942:u8)
            n385 = Increment(x=w943) -> (x+1=w945:i32)
          }
        }
        n386 = Build Array(w931) -> (w936:u8[])
        n387 = Bundle By Name(cluster=w927, "Current Read Index"=w930, "CRCRead"=w936) -> (w926:T6)
        n388 = call <vilib>:"Add State(s) to Queue__jki_lib_state_machine.vi"("State(s) in (\"\")"=w939) -> ("States Out"=w938:string)  [unwired: 14 in]
      }
      frame #41 {
        w948 = u8 224  # ESC
        # "Template Separator\n(You can make a copy of, or modify, this frame)"
        n389 = Unbundle By Name(w947) -> ("ReadArray"=w956:u8[], "CRCRead"=w953:u8[], "Current Read Index"=w954:i32)
        n390 = Increment(x=w954) -> (x+1=w955:i32)
        n391 = Index Array(array=w956, index=w954) -> (element=w957:u8)
        n392 = Equal?(x=w957, y=w948) -> (x = y?=w949:bool)
        n393 = case shown="True" w949 {
          tunnel: [w961 w963] -> w951
          tunnel: [w962 w966] -> w950
          tunnel: w956 -> [_ w965]
          tunnel: w955 -> [w962 w964]
          tunnel: w957 -> [w961 _]
          frame #0 {
          }
          frame #1 {
            n394 = Increment(x=w964) -> (x+1=w966:i32)
            n395 = Index Array(array=w965, index=w964) -> (element=w963:u8)
          }
        }
        n396 = Build Array (concatenate)(w953, w951) -> (w952:u8[])
        n397 = Bundle By Name(cluster=w947, "Current Read Index"=w950, "CRCRead"=w952) -> (w946:T6)
        n398 = call <vilib>:"Add State(s) to Queue__jki_lib_state_machine.vi"("State(s) in (\"\")"=w960) -> ("States Out"=w959:string)  [unwired: 14 in]
      }
      frame #42 {
        # "Template Separator\n(You can make a copy of, or modify, this frame)"
        n399 = Unbundle By Name(w972) -> ("CRCRead"=w974:u8[], "CRCArray"=w967:u8[])
        "CRCRead 2" <- w974
        "CRCArray" <- w967
        n400 = local write "DataReturned"(w967) -> ()
        n401 = call "crc16-ccitt (x1021).vi"("error in (no error)"=w970, "unsigned byte array"=w967) -> ("error out (dup)"=w969:errorcluster, "CRC"=w973:u8[])  [unwired: 8 in]
        "CRC Calc" <- w973
        n402 = Equal?(x=w974, y=w973) -> (x = y?=w968:bool)
        n403 = local write "CRC Match"(w968) -> ()
        n404 = Bundle By Name(cluster=w972, "CRC"=w968) -> (w971:T6)
        n405 = call <vilib>:"Add State(s) to Queue__jki_lib_state_machine.vi"("State(s) in (\"\")"=w976) -> ("States Out"=w975:string)  [unwired: 14 in]
      }
      frame #43 {
        w987 = u8 227  # ETX
        # "Template Separator\n(You can make a copy of, or modify, this frame)"
        n406 = Unbundle By Name(w981) -> ("ReadArray"=w983:u8[], "Current Read Index"=w986:i32)
        n407 = Index Array(array=w983, index=w986) -> (element=w984:u8)
        n408 = Increment(x=w986) -> (x+1=w985:i32)
        n409 = Equal?(x=w984, y=w987) -> (x = y?=w982:bool)
        n410 = case shown="False" w982 {
          tunnel: w979 -> [w993 w995]
          tunnel: [w990 w995] -> w978
          tunnel: ["Exit" ("State(s) in Front (\"\")") _] -> w977
          frame #0 {
            n411 = call "Error Bool Enumerator.vi"("Error Enum"=HEWH_Error_Enumeration."GEA2 ETX", "Error In"=w993, "Error?"=TRUE) -> ("Error Out"=w990:errorcluster)  [unwired: 6 in]
          }
          frame #1 {
          }
        }
        n412 = Bundle By Name(cluster=w981, "Current Read Index"=w985) -> (w980:T6)
        n413 = call <vilib>:"Add State(s) to Queue__jki_lib_state_machine.vi"("State(s) in Front (\"\")"=w977, "State(s) in (\"\")"=w989) -> ("States Out"=w988:string)  [unwired: 13 in]
      }
    }
    n414 = flat-sequence {
      tunnel: [w49] -> w36
      tunnel: w37 -> [_]
      tunnel: [w48] -> w35
      frame #0 {
        n415 = local read "tStart"() -> (w48:u32)
        n416 = Tick Count (ms)() -> (millisecond timer value=w49:u32)
      }
    }
    n417 = Build Array (concatenate)(w32, w31) -> (w30:string[])
    "State Array" <- w30
    n418 = local write "Error Out"(w37) -> ()
    n419 = To Long Integer(number=w36) -> (32bit integer=w34:i32)
    n420 = To Long Integer(number=w35) -> (32bit integer=w33:i32)
  }
  n421 = Subtract(x=w10, y=w9) -> (x-y=w11:i32[])
  "Time Array" <- w11
  n422 = Unbundle By Name(w3) -> ("ReadArray"=w1:u8[], "CRC"=w4:bool)
  n423 = Delete From Array(array=w11, length=1, index=0) -> (array with subset deleted=w13:i32[])  [unwired: 1 out]
  n424 = Unbundle By Name(w3) -> ("Error Out Flag"=w2:bool)
  n425 = for {
    tunnel: w13 -> [w998] mode=indexing
    tunnel: w11 -> [w997] mode=indexing
    tunnel: [w996] -> w12 mode=indexing
    n426 = Subtract(x=w998, y=w997) -> (x-y=w996:i32)
  }
  "Tdiff" <- w12
  n427 = local write "ReadArray"(w1) -> ()
  n428 = Bundle By Name(cluster=w16, "status"=w2) -> (w5:errorcluster)
  n429 = disable-structure shown="Enabled" {
    disable-tunnel: [w1013 w1017] -> w6
    disable-tunnel: w5 -> [w1012 w1017]
    disable-tunnel: w4 -> [w1011 _]
    frame #0 {
      # "Patch for double read of ICP"
      n430 = call "Error Bool Enumerator.vi"("Error Enum"=HEWH_Error_Enumeration."GEA2 Send ACK Mismatch", "Error?"=TRUE) -> ("Error Out"=w1000:errorcluster)  [unwired: 7 in]
      n431 = call "Error Bool Enumerator.vi"("Error Enum"=HEWH_Error_Enumeration."GEA2 ETX", "Error?"=TRUE) -> ("Error Out"=w1002:errorcluster)  [unwired: 7 in]
      n432 = Unbundle By Name(w1000) -> ("code"=w999:i32)
      n433 = Unbundle By Name(w1002) -> ("code"=w1001:i32)
      n434 = Unbundle By Name(w1012) -> ("code"=w1008:i32)
      n435 = Equal?(x=w1008, y=w1001) -> (x = y?=w1009:bool)
      n436 = Equal?(x=w1008, y=w999) -> (x = y?=w1007:bool)
      n437 = Or(x=w1009, y=w1007) -> (x .or. y?=w1010:bool)
      n438 = And(x=w1011, y=w1010) -> (x .and. y?=w1014:bool)
      n439 = case shown="True" w1014 {
        tunnel: [w1015 errorcluster {"status"=FALSE, "code"=0, "source"="ETX or ACK"} ("Error Out")] -> w1013
        tunnel: w1012 -> [w1015 _]
        frame #0 {
        }
        frame #1 {
        }
      }
    }
    frame #1 {
    }
  }
  "Error Out" <- w6
